vi "Main.vi"() -> ()   [LabVIEW 2020]
doc: "This Continuous Measurement sample project is based on the Queued Message Handler template.\n\nThe Event Handling Loop generates messages based on user interface actions.\n\nThe Message Handling Loop processes messages generated by the Event Handling Loop, or by other messages. There are also Acquisition and Logging message handling loop subVIs, and a chart updating loop."
uses:
  controls/UI Data.ctl
  Modbus/Modbus All Data.ctl
  Modbus/Modbus PLC Data All.ctl
  Modbus/Modbus FVIR Control.ctl
  Modbus/Modbus LDO Control.ctl
  WritingDataFile/Data to Save.ctl
  Modbus/Modbus Gas Meter Data.ctl
  Drivers/Alicat LabVIEW Drivers 2v1/Sub-VIs/Data Cluster.ctl
  Drivers/Alicat LabVIEW Drivers 2v1/Sub-VIs/Units of Measure.ctl
  Drivers/Inficon Transmitter/Type Definitions/Inficon Data.ctl
  support/Event Booleans.ctl
  support/Message Queue/Enqueue Message (Single).vi
  <vilib>/Utility/error.llb/Error Cluster From Error Code.vi
  <vilib>/ErrorRing/Error Ring.xnode
  support/User Event - Stop/User Event - Stop.lvlib
  support/Message Queue/Message Queue.lvlib
  Modbus/Modbus.lvlib
  ReadingDataFile/ReadingDataFile.lvlib
  WritingDataFile/WritingDataFile.lvlib
panel:
  out "Message Loop":string[](array[string])
  out "Numeric 2":i32
  out "Numeric":i32
  in  "Tab Control":enum32{"FVIR", "LDO", "Administrator"}(tab)
  out "Actuator spill can is going to Work Pos - FVIR":bool
  out "Actuator spill can is going to Home Pos - FVIR":bool
  out "Actuator mannequin is going to Work Pos - FVIR":bool
  out "Actuator mannequin is going to Home Pos - FVIR":bool
  out "Error - FVIR":bool caption="Error"
  out "Status for error - FVIR":string caption="Error status for FVIR"
  in  "Move mannequin - Go to Work Pos":bool
  in  "Move mannequin - Go to Home Pos":bool
  in  "Spill can - Go to Work Pos":bool
  in  "Spill can - Go to Home Pos":bool
  out "Start recording data - FVIR":bool
  out "Test chamber is in sequence - FVIR":bool
  out "Can is spilling - FVIR":bool
  out "Mannequin is moving - FVIR":bool
  in  "Select test case":i32(listbox)
  in  "Stop Test Case FVIR":bool
  in  "Start Test Case FVIR":bool
  in  "Time Delay of Change direction of Mannequin Actuators":u16=1000
  in  "Number of Mannequin Movement":u16=3
  in  "Water Outlet Proportional Valve EPV-312B":u16=3
  in  "Water Temperature Intellifaucet DRK375":u16=70
  in  "Water Flow Intellifaucet DRK375":u16=15
  in  "Time Pause Between Next Mannequin Sequence":u16=60
  in  "Send parameters to PLC FVIR":bool
  in  "Water Outlet Valve Close FVIR":bool
  in  "Water Outlet Valve Open FVIR":bool
  in  "Gas Solenoid Valve Close FVIR":bool
  in  "Gas Solenoid Valve Open FVIR":bool
  in  "Water Inlet Valve Close FVIR":bool
  in  "Water Inlet Valve Open FVIR":bool
  in  "Water Flow Intellifaucet DRK375 Close FVIR":bool
  in  "Water Flow Intellifaucet DRK375 Open FVIR":bool
  out "Temperatures - FVIR":string[][](array[string])
  out "Sensors - FVIR":string[][](array[string])
  in  "Water Outlet Flow Proportional Valve EPV-312B Close FVIR":bool
  in  "Water Outlet Flow Proportional Valve EPV-312B Open FVIR":bool
  out "Water Outlet Flow Proportional - FVIR":bool
  out "Water flow DRK375 is open - FVIR":bool
  out "Gas Solenoid Valuce - FVIR":bool
  out "Water Inlet Valve - FVIR":bool
  out "Water Outlet Valve - FVIR":bool
  out "General status for FVIR":string
  out "Higher than 1.8% butane":bool
  in  "Start":bool
  in  "Stop":bool
  in  "Path to local logfile":path=path "C:/Users/christian.hansen/Desktop/GE Appliance - FVIR/GEA_Labview_FVIR/CH1234dummy.LOG"
  in  "Reset Flow Meter":bool
  in  "Gas Meter Tare Total":bool
  in  "Gas Meter Tare Rate":bool
  out "Data":string[][](array[string])
  in  "Proportioning Valve":dbl(slide) max=100.0 scale=0.0..100.0
  in  "Valve % Open":dbl(slide)=15.0 min=15.0 max=100.0 scale=15.0..100.0
  in  "Temp (°F)":dbl(slide)=32.0 min=32.0 max=203.0 scale=32.0..200.0
  in  "Water Flow Intellifaucet DRK375 Open LDO":bool
  in  "Water Flow Intellifaucet DRK375 Close LDO":bool
  out "Heater ON/OFF - LDO":bool
  out "Oil spray 1.33cc/min - LDO":bool
  out "Oil spray 1.1cc/min - LDO":bool
  out "Oil spray 0.8cc/min - LDO":bool
  out "Burner ON":bool
  out "Start recording data - LDO":bool
  out "Test chamber is in sequence - LDO":bool
  in  "Stop Test Case LDO":bool
  in  "Start Test Case LDO":bool
  in  "Water Outlet Valve Close LDO":bool
  in  "Water Outlet Valve Open LDO":bool
  in  "Water Inlet Valve Close LDO":bool
  in  "Water Inlet Valve Open LDO":bool
  in  "Gas Solenoid Valve Close LDO":bool
  in  "Gas Solenoid Valve Open LDO":bool
  in  "Oil Spray 0.8 cc/min Close":bool
  in  "Oil Spray 0.8 cc/min Open":bool
  in  "Oil Spray 1.1 cc/min Close":bool
  in  "Oil Spray 1.1 cc/min Open":bool
  in  "Oil Spray 1.33 cc/min Close":bool
  in  "Oil Spray 1.33 cc/min Open":bool
  in  "Heater OFF":bool
  in  "Heater ON":bool
  out "Water Outlet Flow Proportional - LDO":bool
  out "Water flow DRK375 is open - LDO":bool
  out "Gas Solenoid Valuce - LDO":bool
  out "Water Inlet Valve - LDO":bool
  out "Water Outlet Valve - LDO":bool
  in  "Temp/Flow PID Selector":bool=TRUE
  in  "Precondition Purge Gallons":u16=200 caption="Precondition Purge Time (Sec)"
  in  "Output Flow Rate Target (Automated Test)":dbl=0.75 caption="Output Flow Target (Automated Test)"
  in  "Pilot Rate (BTU/hr)":dbl=600.0
  in  "Output Temperature Target (Automated Test)":dbl=135.0
  out "FVIR PLC lifebit":bool
  out "Labview lifebit":bool
  in  "Send parameters to PLC LDO":bool
  in  "Burner cycle 1 to 10 - Duty cycle ON (default 55 min.)":u16=55 caption="Burner cycle 1 to 10 - Duty cycle ON"
  in  "Burner cycle 1 to 10 - Duty cycle OFF (default 5 min.)":u16=5 caption="Burner cycle 1 to 10 - Duty cycle OFF"
  in  "Burner cycle 11 to 12 - Duty cycle ON (default 235 min.)":u16=235 caption="Burner cycle 11 to 12 - Duty cycle ON"
  in  "Burner cycle 11 to 12 - Duty cycle OFF (default 5 min.)":u16=5 caption="Burner cycle 11 to 12 - Duty cycle OFF"
  in  "Burner cycle 13 to end - Duty cycle ON (default 55 min.)":u16=55 caption="Burner cycle 13 to end - Duty cycle ON"
  in  "Burner cycle 13 to end - Duty cycle OFF (default 5 min.)":u16=5 caption="Burner cycle 13 to end - Duty cycle OFF"
  in  "Oil 1st sequence ON (default 5 min.)":u16=5 caption="Oil 1st sequence ON"
  in  "Oil 1st sequence OFF (default 5 min.)":u16=25 caption="Oil 1st sequence OFF"
  in  "All subsequent sequence ON (default 3 min.)":u16=3 caption="All subsequent sequence ON"
  in  "All subsequent sequence OFF (default 27 min.)":u16=27 caption="All subsequent sequence OFF"
  in  "Oil spray preconditioning period ON (default 10 min.)":u16=10 caption="Oil spray preconditioning period ON"
  in  "Oil spray preconditioning period OFF  (default 20 min.)":u16=20 caption="Oil spray preconditioning period OFF"
  out "General status for LDO":string
  out "Status for error - LDO":string caption="Error status for LDO"
  out "Error - LDO":bool caption="Error"
  in  "PLC IP address":string="10.2.0.11"
  in  "Inficon IP Address":string="192.168.1.32"
  in  "Ultramat 23":refnum<visa-resource-name>="COM13"
  # "FVIR and LDO:Swap the data, i.e. 28-10-2021 --> 2021-10-28. --> Lets test this first to see the currents PC timeformat. \nAll data is in the file now. Also the status of LEDs and what Labview is sending --> A lot of redundant info here. What from \nLabview --> PLC should be recorded?"
  # "FVIR: Missing implementation: Getting the glas flow rate, SQRH. CO, CO2 and O2 from the VI's from GEA"
  # "FVIR"
  # "Main control"
  # "Actuator spill can is going to Work Pos"
  # "Actuator spill can is going to Home Pos"
  # "Actuator mannequin is going to Work Pos"
  # "Actuator mannequin is going to Home Pos"
  # "Automatic mode"
  # "Start recording FVIR data"
  # "Test chamber is in sequence"
  # "Can is spilling"
  # "Mannequin is moving"
  # "Water Outlet Valve"
  # "Gas Solenoid Valve"
  # "Water Inlet Valve"
  # "Water Flow Intellifaucet DRK375"
  # "Water Outlet Flow Proportional EPV-312B"
  # "Water Outlet Flow Proportional is open"
  # "Water flow DRK375 is open"
  # "Gas Solenoid is open"
  # "Water Inlet is open"
  # "Water Outlet is open"
  # "Status of valves"
  # "Manual mode"
  # "Temperature from textfile - 4 channels"
  # "Status of actuators"
  # "Values from FVIR sensors"
  # "Status of chamber"
  # "Changing parameters to PLC"
  # "Main control"
  # "Manual mode"
  # "Status of devices"
  # "Status of chamber"
  # "Status of valves"
  # "Water Flow Intellifaucet DRK375"
  # "Gas Meter"
  # "Rotary Actuator"
  # "Oil spray 1.33cc/min"
  # "Oil spray 1.1cc/min"
  # "Oil spray 0.8cc/min"
  # "Start recording LDO data"
  # "Test chamber is in sequence"
  # "Automatic mode"
  # "Start and stop LDO test"
  # "Water Outlet Valve"
  # "Water Inlet Valve"
  # "Gas Solenoid Valve"
  # "Oil spray at 0.8 cc/min"
  # "Oil spray at 1.1 cc/min"
  # "Oil spray at 1.33 cc/min"
  # "Heater"
  # "Water Outlet Flow Proportional is open"
  # "Water flow DRK375 is open"
  # "Gas Solenoid is open"
  # "Water Inlet is open"
  # "Water Outlet is open"
  # "LDO Parameters -"
  # "Changing parameters to PLC"
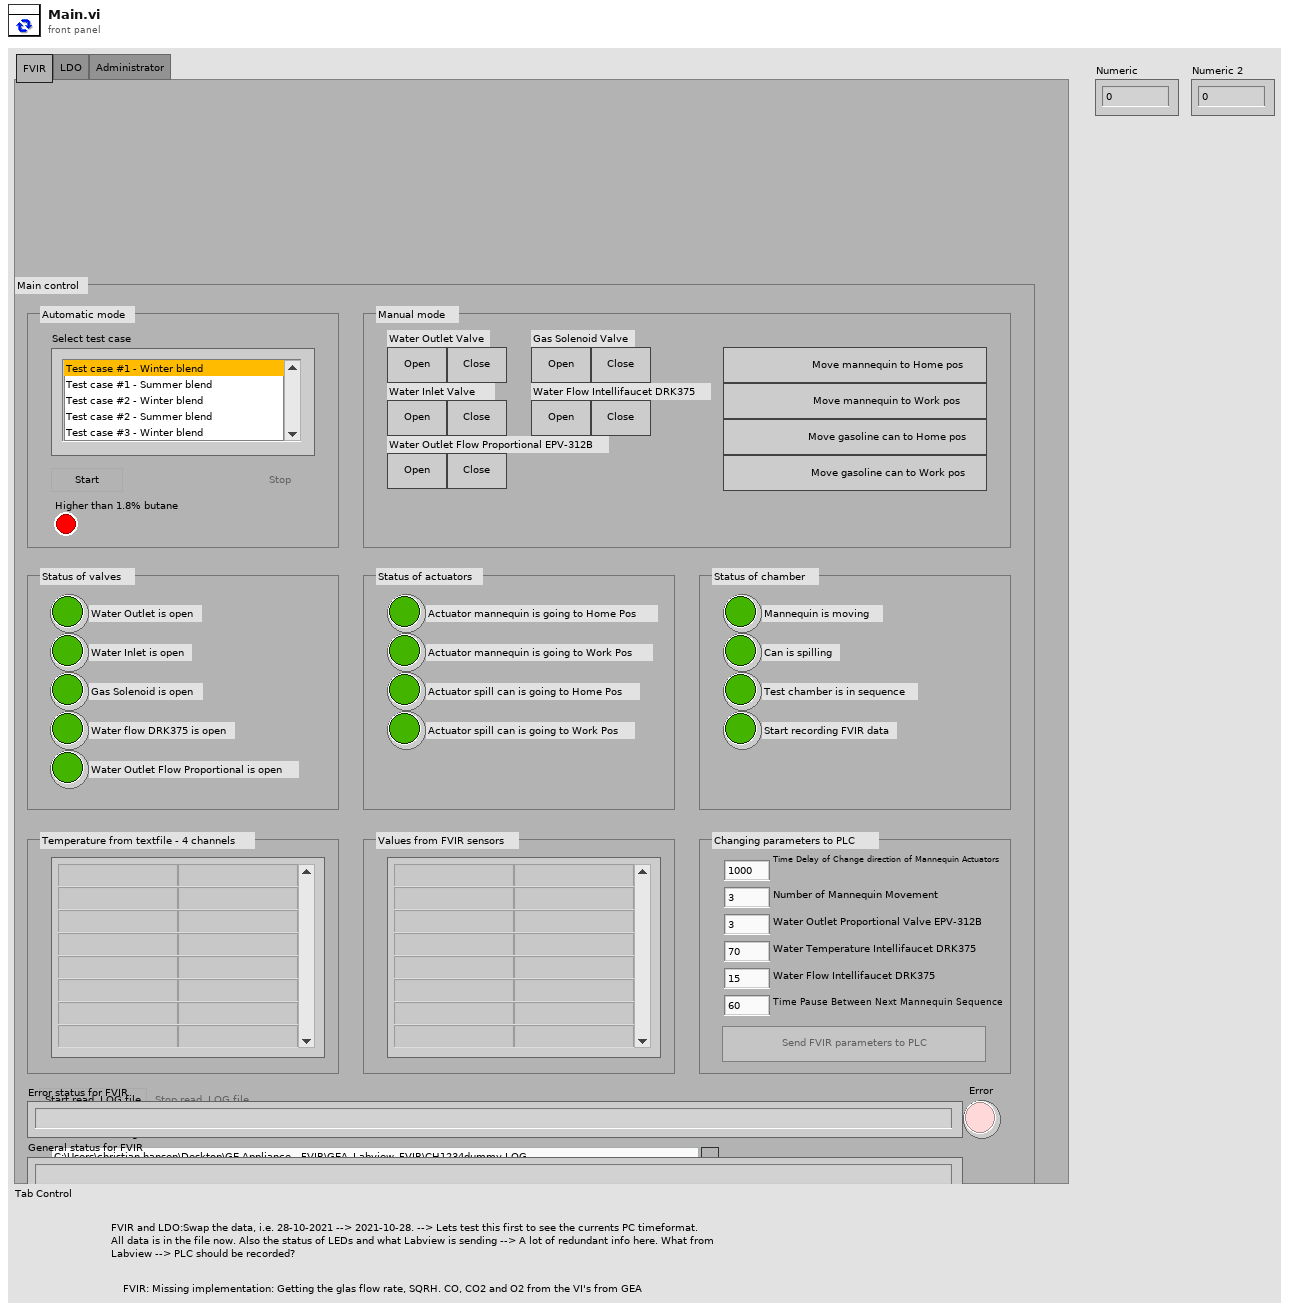
[diagram p1: front panel]
types:
  T1 = typedef "Event Booleans.ctl" = cluster{"Burner ON":bool, "0.8 ml Bool":bool, "1.1 Bool":bool, "1.33 Bool":bool}
  T2 = typedef "Modbus All Data.ctl" = cluster{"PLC Data Out":T3, "Gas Data":T7, "Inficon Data Input":T10, "Ultramat 23":string[][]}
  T3 = typedef "Modbus PLC Data All.ctl" = cluster{"FVIR Data Input":T4, "LDO Control Input":T5, "PLC Input Registers":u16[], "Data to Save":T6}
  T4 = typedef "Modbus FVIR Control.ctl" = cluster{"Spare 15":bool, "Spare 14":bool, "Actuator mannequin is going to Work Pos - FVIR":bool, "Actuator mannequin is going to Home Pos - FVIR":bool, "Test chamber is in sequence - FVIR ":bool, "Water flow DRK375 is open - FVIR":bool, "Gas Solenoid Valve - FVIR":bool, "Water Inlet Valve - FVIR":bool, "Water Outlet Flow Proportional - FVIR":bool, "Start recording data - FVIR":bool, "Actuator spill can is going to Work Pos - FVIR":bool, "Actuator spill can is going to Home Pos - FVIR":bool, "Water Outlet Valve - FVIR":bool, "Can is spilling - FVIR":bool, "Mannequin is moving - FVIR":bool, "FVIR PLC lifebit":bool, "Status for Error - FVIR":string, "Error-FVIR":bool, "Sensors -FVIR":string[][]}
  T5 = typedef "Modbus LDO Control.ctl" = cluster{"LDO PLC Life Bit":bool, "Start recording data - LDO":bool, "Spare 1":bool, "Water Outlet Valve - LDO":bool, "Water Inlet Valve - LDO":bool, "Gas Solenoid Valve - LDO":bool, "Water flow DRK375 is open - LDO":bool, "Test chamber is in sequence - LDO":bool, "Oil spray 0.8cc/min - LDO":bool, "Oil spray 1.1cc/min - LDO":bool, "Oil spray 1.33cc/min - LDO":bool, "Heater ON/OFF - LDO":bool, "Water Outlet Flow Proportional - LDO":bool, "Spare 2":bool, "Spare 3":bool, "Spare 4":bool, "Status for error - LDO":string, "Error - LDO":bool, "Sensor Data":string[][]}
  T6 = typedef "Data to Save.ctl" = cluster{"LDO Full Data":string[][], "FVIR Full Data":string[][], "Test Case - FVIR":string, "Test Case - LDO":string}
  T7 = typedef "Modbus Gas Meter Data.ctl" = cluster{"Data Cluster":T8, "Units of Measure Input":T9, "Header Array":string[]}
  T8 = typedef "Data Cluster.ctl" = cluster{"Absolute Pressure":dbl, "Gauge/Diff. Pressure":dbl, "Barometric Pressure":dbl, "Temperature":dbl, "Volumetric Flow":dbl, "Mass Flow":dbl, "Setpoint":dbl, "Valve Drive":dbl, "Totalizer":dbl, "[hr]":dbl, "[min]":dbl, "[sec]":dbl, "Totalizer Average Flow":dbl, "Totalizer Peak Flow":dbl, "Gas selected":string}
  T9 = typedef "Units of Measure.ctl" = cluster{"Abs. Pressure":string, "Gauge/Diff. Press.":string, "Barometric Press.":string, "Temperature":string, "Volume":string, "Mass":string, "Setpoint":string, "Valve Drive":string, "Totalizer":string, "Tot. Timer":string, "Tot. Avg. Flow":string, "Tot. Peak Flow":string}
  T10 = typedef "Inficon Data.ctl" = cluster{"Gross Heating Value, Vol (Real, Dry)":dbl, "Nitrogen Component Normalized Mole % (Dry)":dbl, "Methane Component Normalized Mole % (Dry)":dbl, "Carbon Dioxide Component Normalized Mole % (Dry)":dbl, "Ethane Component Normalized Mole % (Dry)":dbl, "Propane Component Normalized Mole % (Dry)":dbl, "i-Pentane Component Normalized Mole % (Dry)":dbl, "i-Butane Component Normalized Mole % (Dry)":dbl, "n-Butane Component Normalized Mole % (Dry)":dbl, "n-Pentane Component Normalized Mole % (Dry)":dbl, "Hexane Component Normalized Mole % (Dry)":dbl, "Heptane Component Normalized Mole % (Dry)":dbl, "Gross Wobbe Index, Real(Dry)":dbl, "Relative Density, Real(Dry)":dbl, "Propylene Component Normalized Mole % (Dry)":dbl, "C4 Olefins Component Normalized Mole % (Dry)":dbl, "Water Component Normalized Mole % (Dry)":dbl}
  T11 = typedef "UI Data.ctl" = cluster{"Start Ref":refnum<vi>, "Stop Ref":refnum<vi>, "Exit Ref":refnum<vi>, "Status Ref":refnum<vi>, "Connect Ref":refnum<vi>, "Disconnect Ref":refnum<vi>, "Spill can Home pos Ref":refnum<vi>, "Spill can Work pos Ref":refnum<vi>, "Move Mannequin Home pos Ref":refnum<vi>, "Move Mannequin Work pos Ref":refnum<vi>, "Start test case FVIR Ref":refnum<vi>, "Water Outlet Valve Open FVIR Ref":refnum<vi>, "Water Inlet Valve Open FVIR Ref":refnum<vi>, "Gas Solenoid Valve Open FVIR Ref":refnum<vi>, "Water Flow Open FVIR Ref":refnum<vi>, "Listbox Ref":refnum<vi>, "Stop test case FVIR Ref":refnum<vi>, "Water Outlet Valve Close FVIR Ref":refnum<vi>, "Water Inlet Valve Close FVIR Ref":refnum<vi>, "Gas Solenoid Valve Close FVIR Ref":refnum<vi>, "Water Flow Close FVIR Ref":refnum<vi>, "Send Param to PLC FVIR Ref":refnum<vi>, "Water Flow Prop Open FVIR Ref":refnum<vi>, "Water Flow Prop Close FVIR Ref":refnum<vi>, "Start test case LDO Ref":refnum<vi>, "Stop test case LDO Ref":refnum<vi>, "Water Outlet Valve Open LDO Ref":refnum<vi>, "Water Outlet Valve Close LDO Ref":refnum<vi>, "Water Inlet Valve Open LDO Ref":refnum<vi>, "Water Inlet Valve Close LDO Ref":refnum<vi>, "Gas Solenoid Valve Open LDO Ref":refnum<vi>, "Gas Solenoid Valve Close LDO Ref":refnum<vi>, "Water Flow Open LDO Ref":refnum<vi>, "Water Flow Close LDO Ref":refnum<vi>, "Water Flow Prop Open LDO Ref":refnum<vi>, "Water Flow Prop Close LDO Ref":refnum<vi>, "Oil spray 0.8cc/min Open Ref":refnum<vi>, "Oil spray 0.8cc/min Close Ref":refnum<vi>, "Oil spray 1.1cc/min Open Ref":refnum<vi>, "Oil spray 1.1cc/min Close Ref":refnum<vi>, "Oil spray 1.33cc/min Open Ref":refnum<vi>, "Oil spray 1.33cc/min Close Ref":refnum<vi>, "Heater ON Ref":refnum<vi>, "Heater OFF Ref":refnum<vi>, "Send Param to PLC LDO Ref":refnum<vi>}
  T12 = typedef "Message Queue.lvlib/All Message Queues.ctl" = cluster{"UI":refnum<queue>, "Modbus":refnum<queue>, "Watchdog":refnum<queue>, "ReadDataFile":refnum<queue>, "DataScanning":refnum<queue>, "WriteDataFile":refnum<queue>, "WatchdogWriteFile":refnum<queue>, "OilMachine":refnum<queue>, "Alicat_GasMeter":refnum<queue>, "Inficon":refnum<queue>, "Ultramat 23":refnum<queue>}
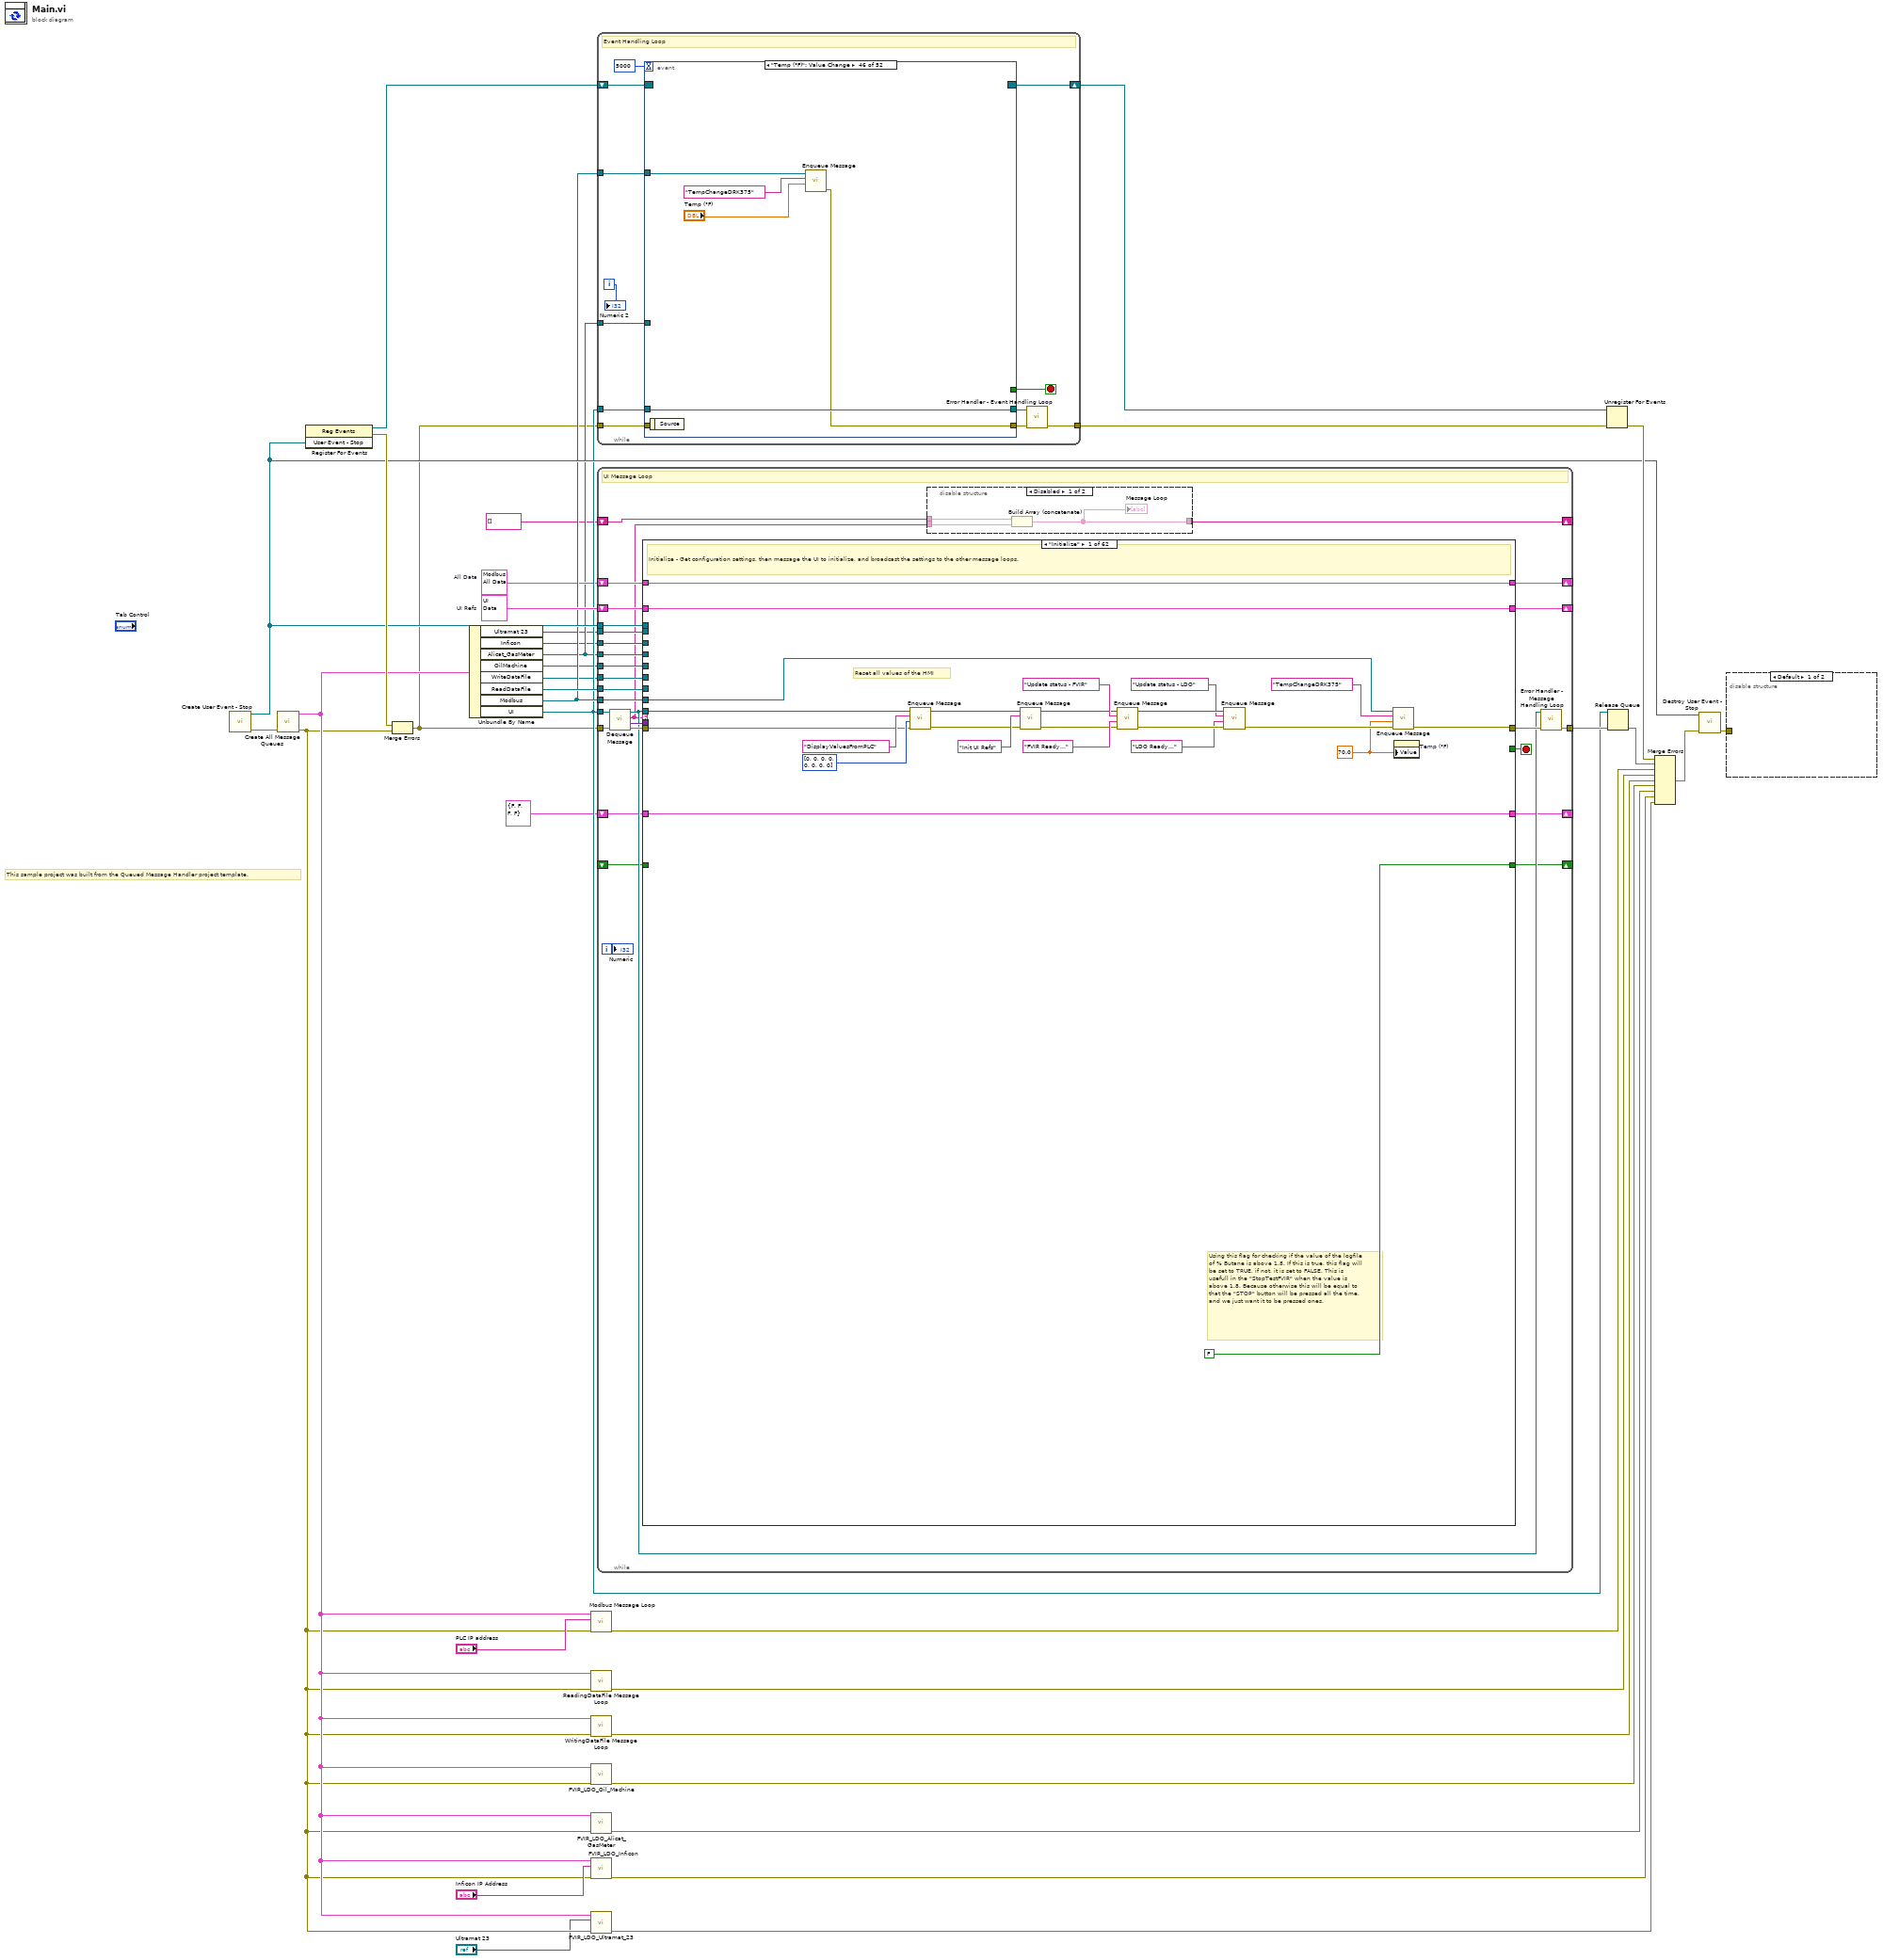
[diagram p0: block diagram]
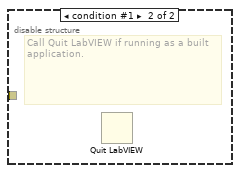
[diagram p2: hidden frame]
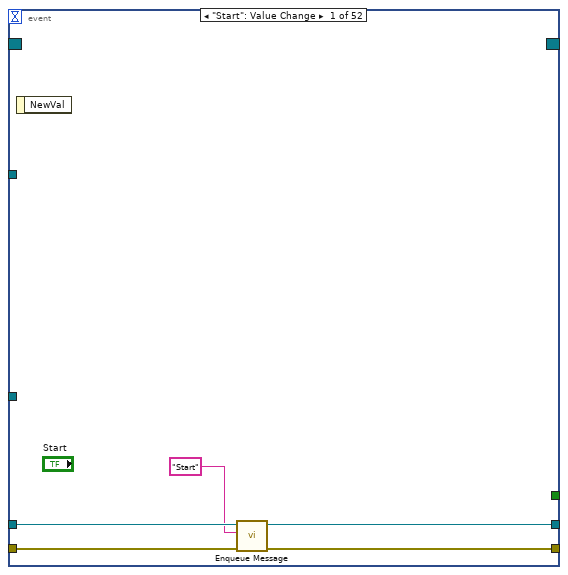
[diagram p3: hidden frame]
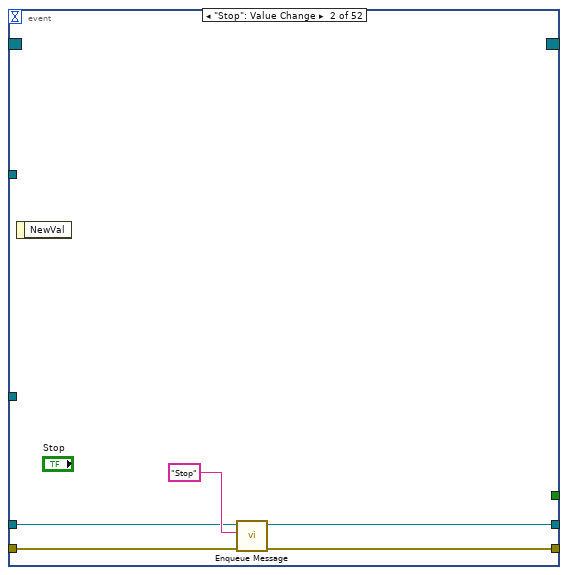
[diagram p4: hidden frame]
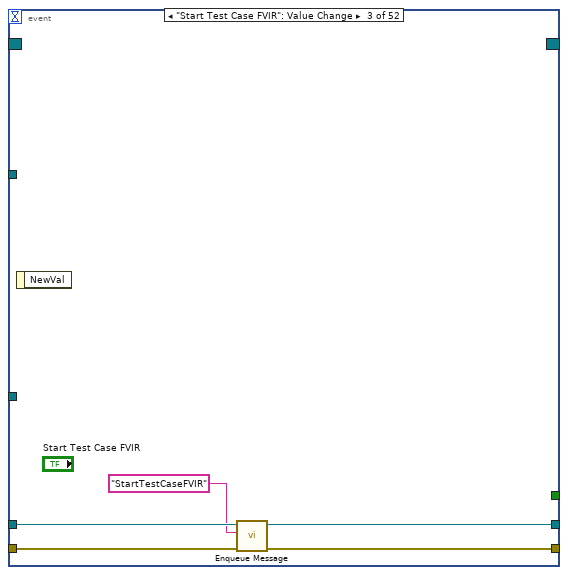
[diagram p5: hidden frame]
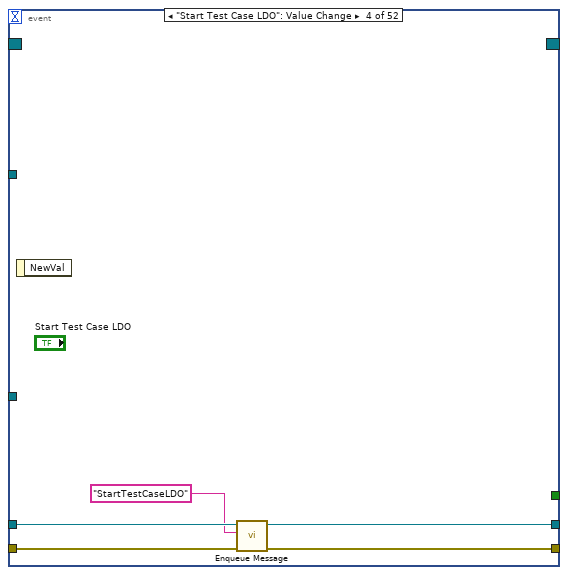
[diagram p6: hidden frame]
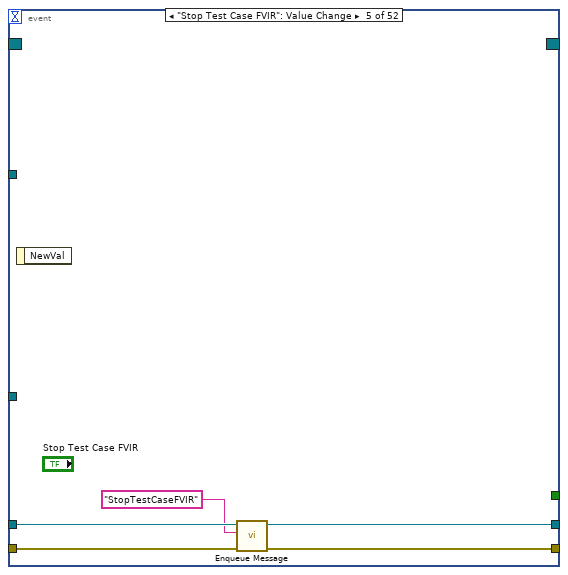
[diagram p7: hidden frame]
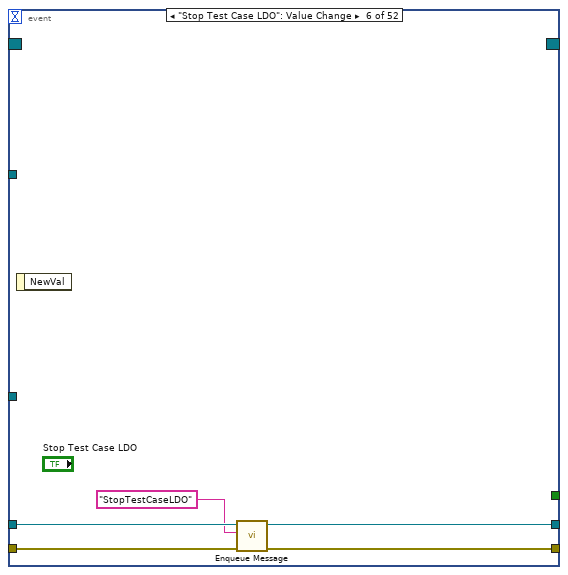
[diagram p8: hidden frame]
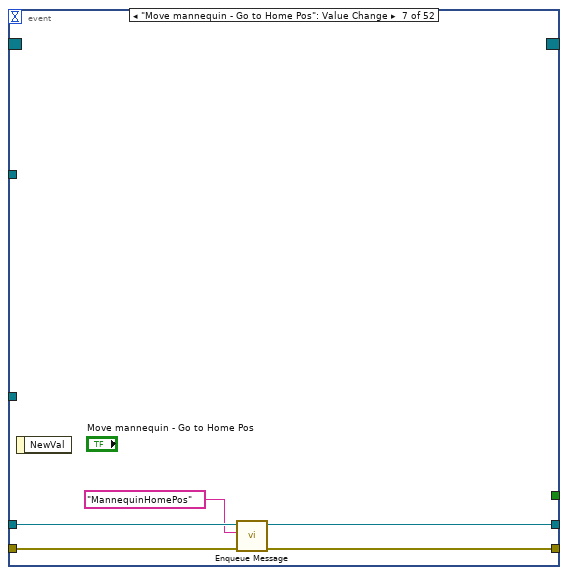
[diagram p9: hidden frame]
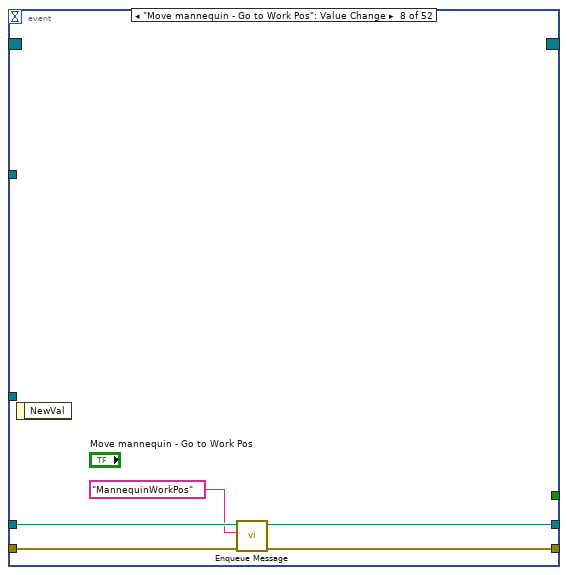
[diagram p10: hidden frame]
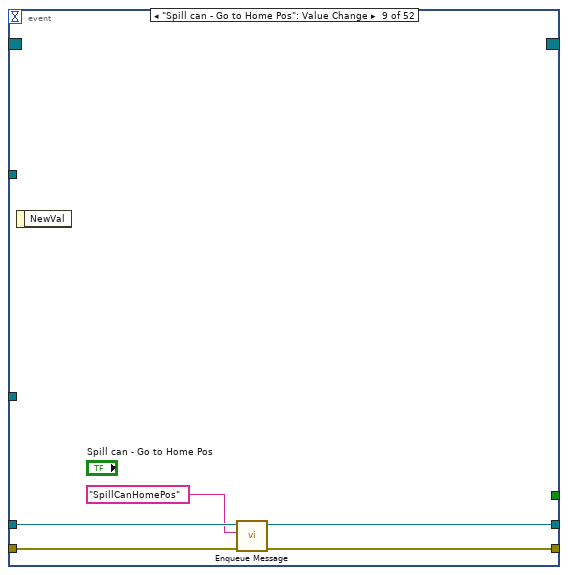
[diagram p11: hidden frame]
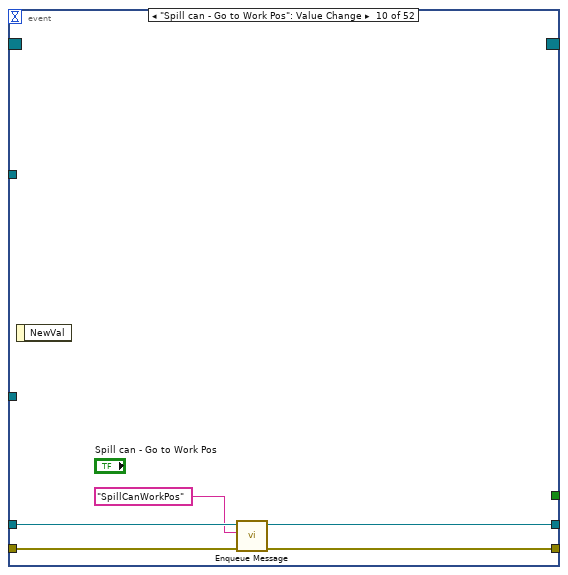
[diagram p12: hidden frame]
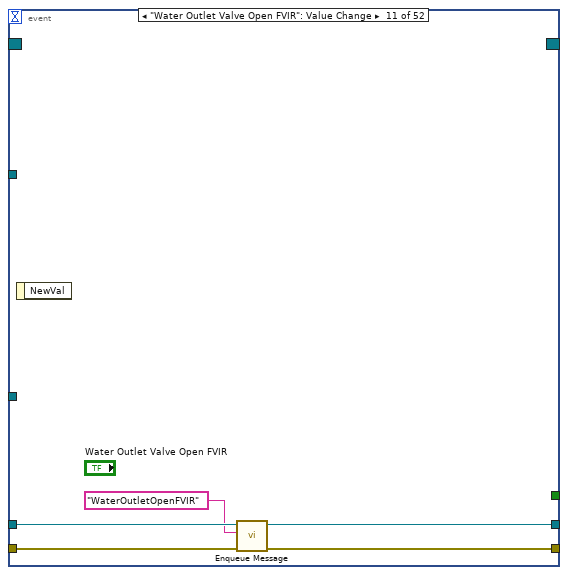
[diagram p13: hidden frame]
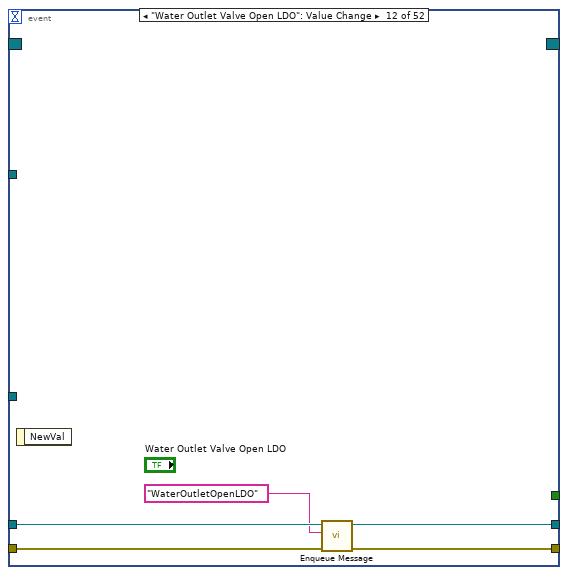
[diagram p14: hidden frame]
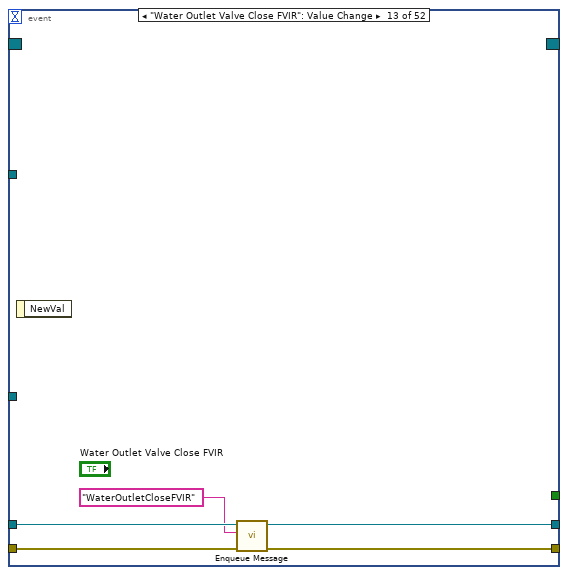
[diagram p15: hidden frame]
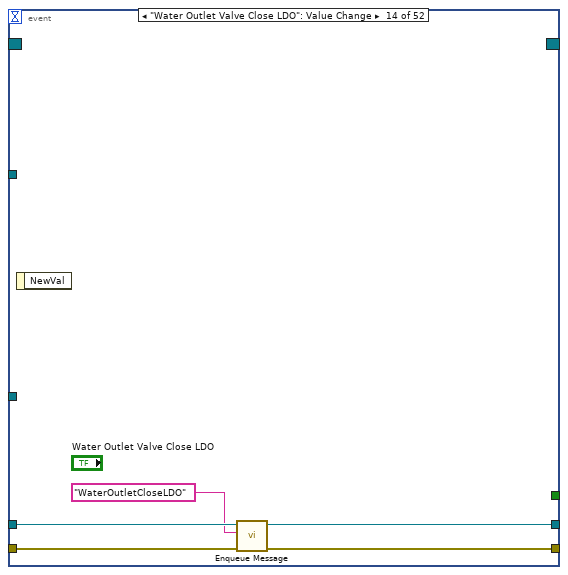
[diagram p16: hidden frame]
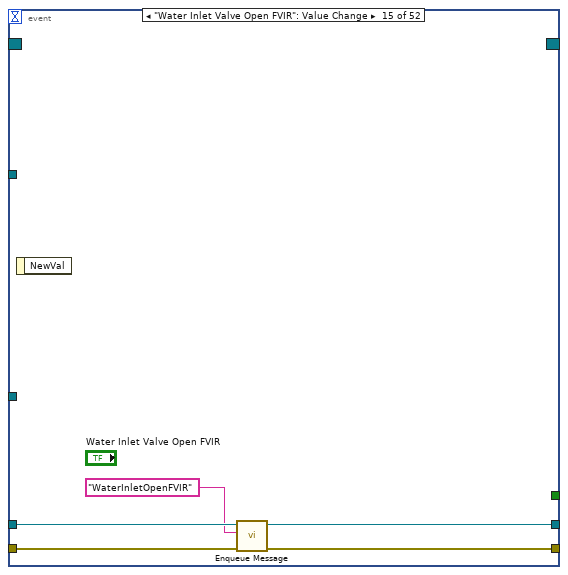
[diagram p17: hidden frame]
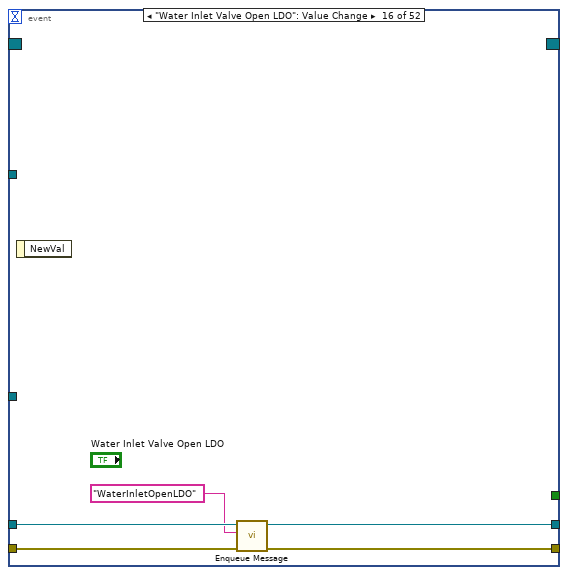
[diagram p18: hidden frame]
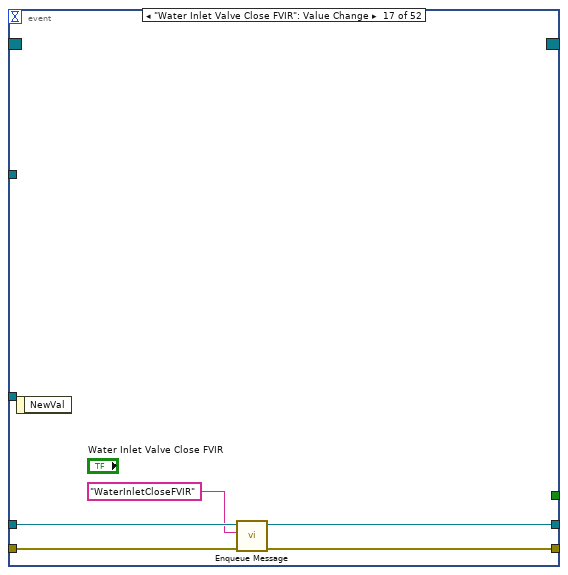
[diagram p19: hidden frame]
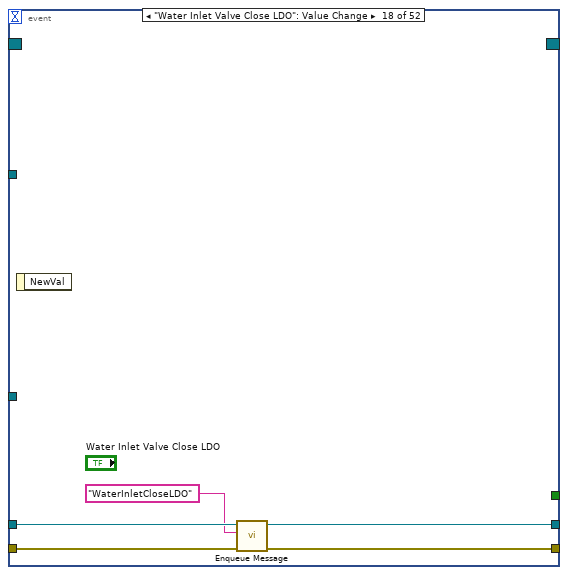
[diagram p20: hidden frame]
diagram:
  w15 = T2 {"PLC Data Out"={"FVIR Data Input"={"Spare 15"=FALSE, "Spare 14"=FALSE, "Actuator mannequin is going to Work Pos - FVIR"=FALSE, "Actuator mannequin is going to Home Pos - FVIR"=FALSE, "Test chamber is in sequence - FVIR "=FALSE, "Water flow DRK375 is open - FVIR"=FALSE, "Gas Solenoid Valve - FVIR"=FALSE, "Water Inlet Valve - FVIR"=FALSE, "Water Outlet Flow Proportional - FVIR"=FALSE, "Start recording data - FVIR"=FALSE, "Actuator spill can is going to Work Pos - FVIR"=FALSE, "Actuator spill can is going to Home Pos - FVIR"=FALSE, "Water Outlet Valve - FVIR"=FALSE, "Can is spilling - FVIR"=FALSE, "Mannequin is moving - FVIR"=FALSE, "FVIR PLC lifebit"=FALSE, "Status for Error - FVIR"="", "Error-FVIR"=FALSE, "Sensors -FVIR"=[]}, "LDO Control Input"={"LDO PLC Life Bit"=FALSE, "Start recording data - LDO"=FALSE, "Spare 1"=FALSE, "Water Outlet Valve - LDO"=FALSE, "Water Inlet Valve - LDO"=FALSE, "Gas Solenoid Valve - LDO"=FALSE, "Water flow DRK375 is open - LDO"=FALSE, "Test chamber is in sequence - LDO"=FALSE, "Oil spray 0.8cc/min - LDO"=FALSE, "Oil spray 1.1cc/min - LDO"=FALSE, "Oil spray 1.33cc/min - LDO"=FALSE, "Heater ON/OFF - LDO"=FALSE, "Water Outlet Flow Proportional - LDO"=FALSE, "Spare 2"=FALSE, "Spare 3"=FALSE, "Spare 4"=FALSE, "Status for error - LDO"="", "Error - LDO"=FALSE, "Sensor Data"=[]}, "PLC Input Registers"=[], "Data to Save"={"LDO Full Data"=[], "FVIR Full Data"=[], "Test Case - FVIR"="", "Test Case - LDO"=""}}, "Gas Data"={"Data Cluster"={"Absolute Pressure"=0.0, "Gauge/Diff. Pressure"=0.0, "Barometric Pressure"=0.0, "Temperature"=0.0, "Volumetric Flow"=0.0, "Mass Flow"=0.0, "Setpoint"=0.0, "Valve Drive"=0.0, "Totalizer"=0.0, "[hr]"=0.0, "[min]"=0.0, "[sec]"=0.0, "Totalizer Average Flow"=0.0, "Totalizer Peak Flow"=0.0, "Gas selected"=""}, "Units of Measure Input"={"Abs. Pressure"="", "Gauge/Diff. Press."="", "Barometric Press."="", "Temperature"="", "Volume"="", "Mass"="", "Setpoint"="", "Valve Drive"="", "Totalizer"="", "Tot. Timer"="", "Tot. Avg. Flow"="", "Tot. Peak Flow"=""}, "Header Array"=[]}, "Inficon Data Input"={"Gross Heating Value, Vol (Real, Dry)"=0.0, "Nitrogen Component Normalized Mole % (Dry)"=0.0, "Methane Component Normalized Mole % (Dry)"=0.0, "Carbon Dioxide Component Normalized Mole % (Dry)"=0.0, "Ethane Component Normalized Mole % (Dry)"=0.0, "Propane Component Normalized Mole % (Dry)"=0.0, "i-Pentane Component Normalized Mole % (Dry)"=0.0, "i-Butane Component Normalized Mole % (Dry)"=0.0, "n-Butane Component Normalized Mole % (Dry)"=0.0, "n-Pentane Component Normalized Mole % (Dry)"=0.0, "Hexane Component Normalized Mole % (Dry)"=0.0, "Heptane Component Normalized Mole % (Dry)"=0.0, "Gross Wobbe Index, Real(Dry)"=0.0, "Relative Density, Real(Dry)"=0.0, "Propylene Component Normalized Mole % (Dry)"=0.0, "C4 Olefins Component Normalized Mole % (Dry)"=0.0, "Water Component Normalized Mole % (Dry)"=0.0}, "Ultramat 23"=[]}  # All Data
  w31 = T11 {"Start Ref"=refnum, "Stop Ref"=refnum, "Exit Ref"=refnum, "Status Ref"=refnum, "Connect Ref"=refnum, "Disconnect Ref"=refnum, "Spill can Home pos Ref"=refnum, "Spill can Work pos Ref"=refnum, "Move Mannequin Home pos Ref"=refnum, "Move Mannequin Work pos Ref"=refnum, "Start test case FVIR Ref"=refnum, "Water Outlet Valve Open FVIR Ref"=refnum, "Water Inlet Valve Open FVIR Ref"=refnum, "Gas Solenoid Valve Open FVIR Ref"=refnum, "Water Flow Open FVIR Ref"=refnum, "Listbox Ref"=refnum, "Stop test case FVIR Ref"=refnum, "Water Outlet Valve Close FVIR Ref"=refnum, "Water Inlet Valve Close FVIR Ref"=refnum, "Gas Solenoid Valve Close FVIR Ref"=refnum, "Water Flow Close FVIR Ref"=refnum, "Send Param to PLC FVIR Ref"=refnum, "Water Flow Prop Open FVIR Ref"=refnum, "Water Flow Prop Close FVIR Ref"=refnum, "Start test case LDO Ref"=refnum, "Stop test case LDO Ref"=refnum, "Water Outlet Valve Open LDO Ref"=refnum, "Water Outlet Valve Close LDO Ref"=refnum, "Water Inlet Valve Open LDO Ref"=refnum, "Water Inlet Valve Close LDO Ref"=refnum, "Gas Solenoid Valve Open LDO Ref"=refnum, "Gas Solenoid Valve Close LDO Ref"=refnum, "Water Flow Open LDO Ref"=refnum, "Water Flow Close LDO Ref"=refnum, "Water Flow Prop Open LDO Ref"=refnum, "Water Flow Prop Close LDO Ref"=refnum, "Oil spray 0.8cc/min Open Ref"=refnum, "Oil spray 0.8cc/min Close Ref"=refnum, "Oil spray 1.1cc/min Open Ref"=refnum, "Oil spray 1.1cc/min Close Ref"=refnum, "Oil spray 1.33cc/min Open Ref"=refnum, "Oil spray 1.33cc/min Close Ref"=refnum, "Heater ON Ref"=refnum, "Heater OFF Ref"=refnum, "Send Param to PLC LDO Ref"=refnum}  # UI Refs
  # "This sample project was built from the Queued Message Handler project template."
  n1 = call "Create User Event - Stop.vi"() -> ("error out"=w34:errorcluster, "User Event - Stop"=w26:refnum<user-event>)  [unwired: 10 in]
  n2 = call "Create All Message Queues.vi"("error in (no error)"=w34) -> ("error out"=w10:errorcluster, "Message Queues out"=w11:T12)  [unwired: 9 in]
  n3 = register-events(w26) -> (reference out=w28:refnum<event-registration>, error out=w27:errorcluster)  [unwired: 2 in]
  n4 = Merge Errors(w27, w10) -> (w2:errorcluster)
  n5 = Unbundle By Name(w11) -> ("Ultramat 23"=w5:refnum<queue>, "Inficon"=w13:refnum<queue>, "Alicat_GasMeter"=w14:refnum<queue>, "OilMachine"=w17:refnum<queue>, "WriteDataFile"=w1:refnum<queue>, "ReadDataFile"=w25:refnum<queue>, "Modbus"=w24:refnum<queue>, "UI"=w19:refnum<queue>)
  n6 = call "Modbus Message Loop.vi"("Message Queues in"=w11, "PLC IP address"="PLC IP address", "error in (no error)"=w10) -> ("error out"=w23:errorcluster)  [unwired: 7 in]
  n7 = call "ReadingDataFile Message Loop.vi"("error in (no error)"=w10, "Message Queues"=w11) -> ("error out"=w22:errorcluster)  [unwired: 7 in, 1 out]
  n8 = call "WritingDataFile Message Loop.vi"("error in (no error)"=w10, "Message Queues"=w11) -> ("error out"=w21:errorcluster)  [unwired: 9 in]
  n9 = call "FVIR_LDO_Oil_Machine.vi"("error in"=w10, "Message Queues"=w11) -> ("error out"=w18:errorcluster)  [unwired: 9 in]
  n10 = call "FVIR_LDO_Alicat_GasMeter.vi"("error in"=w10, "Message Queues"=w11) -> ("error out"=w9:errorcluster)  [unwired: 9 in]
  n11 = call "FVIR_LDO_Inficon.vi"("error in"=w10, "Remote IP Address"="Inficon IP Address", "Message Queues"=w11) -> ("error out"=w8:errorcluster)  [unwired: 8 in]
  n12 = call "FVIR_LDO_Ultramat_23.vi"("error in"=w10, "VISA resource name"="Ultramat 23", "Message Queues"=w11) -> ("error out"=w7:errorcluster)  [unwired: 8 in]
  n13 = while {
    tunnel: w19 -> [w47]
    tunnel: [w44] -> w35
    shift-right: [w46] -> w32
    shift-left: w28 -> [w48]
    tunnel: w24 -> [w40]
    tunnel: w14 -> [w39]
    tunnel: w2 -> [w37]
    i -> [w38]
    stop <- w45 stop-if-true
    # "Event Handling Loop"
    n14 = event shown="[45] \"Temp (°F)\": Value Change" {
      selector: w48 -> [_ _ _ _ _ _ _ _ _ _ _ _ _ _ _ _ _ _ _ _ _ _ _ _ _ _ _ _ _ _ _ _ _ _ _ _ _ _ _ _ _ _ _ _ _ _ _ _ _ _ _ _]
      dyn-events: [_ _ _ _ _ _ _ _ _ _ _ _ _ _ _ _ _ _ _ _ _ _ _ _ _ _ _ _ _ _ _ _ _ _ _ _ _ _ _ _ _ _ _ _ _ _ _ _ _ _ _ _] -> w46
      timeout: 5000 -> [_ _ _ _ _ _ _ _ _ _ _ _ _ _ _ _ _ _ _ _ _ _ _ _ _ _ _ _ _ _ _ _ _ _ _ _ _ _ _ _ _ _ _ _ _ _ _ _ _ _ _ _]
      tunnel: [_ _ _ _ _ _ _ _ _ _ _ _ _ _ _ _ _ _ _ _ _ _ _ _ _ _ _ _ _ _ _ _ _ _ _ _ _ _ _ _ _ _ _ TRUE ("Discard?") _ _ _ _ _ _ _ _] -> w45
      tunnel: w47 -> [w53 w57 w63 w68 w73 w78 w83 w88 w93 w98 w103 w108 w113 w118 w123 w128 w133 w138 w143 w148 w153 w158 w163 w173 w180 w190 w197 w202 w207 w212 w217 w225 w230 w235 w243 w248 w253 w261 w266 w271 w276 w281 w285 w288 w291 w308 w313 w318 w322 w326 w335 w342]
      tunnel: [w51 w56 w61 w66 w71 w76 w81 w86 w91 w96 w101 w106 w111 w116 w121 w126 w131 w136 w141 w146 w151 w156 w161 w169 w178 w188 w195 w200 w205 w210 w216 w223 w228 w233 w241 w246 w251 w259 w264 w269 w274 w279 w284 w286 w296 w304 w309 w314 w319 w323 w330 w340] -> w43
      tunnel: [w50 w55 w60 w65 w70 w75 w80 w85 w90 w95 w100 w105 w110 w115 w120 w125 w130 w135 w140 w145 w150 w155 w160 w170 w177 w186 w194 w199 w204 w209 w215 w222 w227 w234 w240 w245 w252 w258 w263 w268 w273 w280 w285 w288 w290 w308 w313 w318 w322 w326 w335 w342] -> w42
      tunnel: w40 -> [_ _ _ _ _ _ _ _ _ _ _ _ _ _ _ _ _ _ _ _ _ _ _ _ _ _ _ _ _ _ _ _ _ _ _ _ _ _ _ _ _ _ _ _ _ w306 w311 w316 _ _ w331 w339]
      tunnel: w39 -> [_ _ _ _ _ _ _ _ _ _ _ _ _ _ _ _ _ _ _ _ _ _ _ _ _ _ _ _ _ _ _ _ _ _ _ _ _ _ _ _ _ _ _ _ _ _ _ _ w320 w324 _ _]
      tunnel: w37 -> [w49 w54 w59 w64 w69 w74 w79 w84 w89 w94 w99 w104 w109 w114 w119 w124 w129 w134 w139 w144 w149 w154 w159 w164 w176 w181 w193 w198 w203 w208 w213 w221 w226 w231 w239 w244 w249 w257 w262 w267 w272 w277 w284 w286 w295 _ _ _ _ _ _ _]
      event "Start": Value Change {
        n15 = event-data() -> ()  [unwired: 1 in, 1 out]
        n16 = call-poly "Enqueue Message.vi"("error in (no error)"=w49, "Message"="Start", "Message Queue"=w53) -> ("error out"=w51:errorcluster, "dup Message Queue"=w50:refnum<queue>)  [unwired: 7 in]
      }
      event "Stop": Value Change {
        n17 = event-data() -> ()  [unwired: 1 in, 1 out]
        n18 = call-poly "Enqueue Message.vi"("error in (no error)"=w54, "Message"="Stop", "Message Queue"=w57) -> ("error out"=w56:errorcluster, "dup Message Queue"=w55:refnum<queue>)  [unwired: 7 in]
      }
      event "Start Test Case FVIR": Value Change {
        n19 = event-data() -> ()  [unwired: 1 in, 1 out]
        n20 = call-poly "Enqueue Message.vi"("error in (no error)"=w59, "Message"="StartTestCaseFVIR", "Message Queue"=w63) -> ("error out"=w61:errorcluster, "dup Message Queue"=w60:refnum<queue>)  [unwired: 7 in]
      }
      event "Start Test Case LDO": Value Change {
        n21 = event-data() -> ()  [unwired: 1 in, 1 out]
        n22 = call-poly "Enqueue Message.vi"("error in (no error)"=w64, "Message"="StartTestCaseLDO", "Message Queue"=w68) -> ("error out"=w66:errorcluster, "dup Message Queue"=w65:refnum<queue>)  [unwired: 7 in]
      }
      event "Stop Test Case FVIR": Value Change {
        n23 = event-data() -> ()  [unwired: 1 in, 1 out]
        n24 = call-poly "Enqueue Message.vi"("error in (no error)"=w69, "Message"="StopTestCaseFVIR", "Message Queue"=w73) -> ("error out"=w71:errorcluster, "dup Message Queue"=w70:refnum<queue>)  [unwired: 7 in]
      }
      event "Stop Test Case LDO": Value Change {
        n25 = event-data() -> ()  [unwired: 1 in, 1 out]
        n26 = call-poly "Enqueue Message.vi"("error in (no error)"=w74, "Message"="StopTestCaseLDO", "Message Queue"=w78) -> ("error out"=w76:errorcluster, "dup Message Queue"=w75:refnum<queue>)  [unwired: 7 in]
      }
      event "Move mannequin - Go to Home Pos": Value Change {
        n27 = event-data() -> ()  [unwired: 1 in, 1 out]
        n28 = call-poly "Enqueue Message.vi"("error in (no error)"=w79, "Message"="MannequinHomePos", "Message Queue"=w83) -> ("error out"=w81:errorcluster, "dup Message Queue"=w80:refnum<queue>)  [unwired: 7 in]
      }
      event "Move mannequin - Go to Work Pos": Value Change {
        n29 = event-data() -> ()  [unwired: 1 in, 1 out]
        n30 = call-poly "Enqueue Message.vi"("error in (no error)"=w84, "Message"="MannequinWorkPos", "Message Queue"=w88) -> ("error out"=w86:errorcluster, "dup Message Queue"=w85:refnum<queue>)  [unwired: 7 in]
      }
      event "Spill can - Go to Home Pos": Value Change {
        n31 = event-data() -> ()  [unwired: 1 in, 1 out]
        n32 = call-poly "Enqueue Message.vi"("error in (no error)"=w89, "Message"="SpillCanHomePos", "Message Queue"=w93) -> ("error out"=w91:errorcluster, "dup Message Queue"=w90:refnum<queue>)  [unwired: 7 in]
      }
      event "Spill can - Go to Work Pos": Value Change {
        n33 = event-data() -> ()  [unwired: 1 in, 1 out]
        n34 = call-poly "Enqueue Message.vi"("error in (no error)"=w94, "Message"="SpillCanWorkPos", "Message Queue"=w98) -> ("error out"=w96:errorcluster, "dup Message Queue"=w95:refnum<queue>)  [unwired: 7 in]
      }
      event "Water Outlet Valve Open FVIR": Value Change {
        n35 = event-data() -> ()  [unwired: 1 in, 1 out]
        n36 = call-poly "Enqueue Message.vi"("error in (no error)"=w99, "Message"="WaterOutletOpenFVIR", "Message Queue"=w103) -> ("error out"=w101:errorcluster, "dup Message Queue"=w100:refnum<queue>)  [unwired: 7 in]
      }
      event "Water Outlet Valve Open LDO": Value Change {
        n37 = event-data() -> ()  [unwired: 1 in, 1 out]
        n38 = call-poly "Enqueue Message.vi"("error in (no error)"=w104, "Message"="WaterOutletOpenLDO", "Message Queue"=w108) -> ("error out"=w106:errorcluster, "dup Message Queue"=w105:refnum<queue>)  [unwired: 7 in]
      }
      event "Water Outlet Valve Close FVIR": Value Change {
        n39 = event-data() -> ()  [unwired: 1 in, 1 out]
        n40 = call-poly "Enqueue Message.vi"("error in (no error)"=w109, "Message"="WaterOutletCloseFVIR", "Message Queue"=w113) -> ("error out"=w111:errorcluster, "dup Message Queue"=w110:refnum<queue>)  [unwired: 7 in]
      }
      event "Water Outlet Valve Close LDO": Value Change {
        n41 = event-data() -> ()  [unwired: 1 in, 1 out]
        n42 = call-poly "Enqueue Message.vi"("error in (no error)"=w114, "Message"="WaterOutletCloseLDO", "Message Queue"=w118) -> ("error out"=w116:errorcluster, "dup Message Queue"=w115:refnum<queue>)  [unwired: 7 in]
      }
      event "Water Inlet Valve Open FVIR": Value Change {
        n43 = event-data() -> ()  [unwired: 1 in, 1 out]
        n44 = call-poly "Enqueue Message.vi"("error in (no error)"=w119, "Message"="WaterInletOpenFVIR", "Message Queue"=w123) -> ("error out"=w121:errorcluster, "dup Message Queue"=w120:refnum<queue>)  [unwired: 7 in]
      }
      event "Water Inlet Valve Open LDO": Value Change {
        n45 = event-data() -> ()  [unwired: 1 in, 1 out]
        n46 = call-poly "Enqueue Message.vi"("error in (no error)"=w124, "Message"="WaterInletOpenLDO", "Message Queue"=w128) -> ("error out"=w126:errorcluster, "dup Message Queue"=w125:refnum<queue>)  [unwired: 7 in]
      }
      event "Water Inlet Valve Close FVIR": Value Change {
        n47 = event-data() -> ()  [unwired: 1 in, 1 out]
        n48 = call-poly "Enqueue Message.vi"("error in (no error)"=w129, "Message"="WaterInletCloseFVIR", "Message Queue"=w133) -> ("error out"=w131:errorcluster, "dup Message Queue"=w130:refnum<queue>)  [unwired: 7 in]
      }
      event "Water Inlet Valve Close LDO": Value Change {
        n49 = event-data() -> ()  [unwired: 1 in, 1 out]
        n50 = call-poly "Enqueue Message.vi"("error in (no error)"=w134, "Message"="WaterInletCloseLDO", "Message Queue"=w138) -> ("error out"=w136:errorcluster, "dup Message Queue"=w135:refnum<queue>)  [unwired: 7 in]
      }
      event "Gas Solenoid Valve Open FVIR": Value Change {
        n51 = event-data() -> ()  [unwired: 1 in, 1 out]
        n52 = call-poly "Enqueue Message.vi"("error in (no error)"=w139, "Message"="GasSolenoidOpenFVIR", "Message Queue"=w143) -> ("error out"=w141:errorcluster, "dup Message Queue"=w140:refnum<queue>)  [unwired: 7 in]
      }
      event "Gas Solenoid Valve Open LDO": Value Change {
        n53 = event-data() -> ()  [unwired: 1 in, 1 out]
        n54 = call-poly "Enqueue Message.vi"("error in (no error)"=w144, "Message"="GasSolenoidOpenLDO", "Message Queue"=w148) -> ("error out"=w146:errorcluster, "dup Message Queue"=w145:refnum<queue>)  [unwired: 7 in]
      }
      event "Gas Solenoid Valve Close FVIR": Value Change {
        n55 = event-data() -> ()  [unwired: 1 in, 1 out]
        n56 = call-poly "Enqueue Message.vi"("error in (no error)"=w149, "Message"="GasSolenoidCloseFVIR", "Message Queue"=w153) -> ("error out"=w151:errorcluster, "dup Message Queue"=w150:refnum<queue>)  [unwired: 7 in]
      }
      event "Gas Solenoid Valve Close LDO": Value Change {
        n57 = event-data() -> ()  [unwired: 1 in, 1 out]
        n58 = call-poly "Enqueue Message.vi"("error in (no error)"=w154, "Message"="GasSolenoidCloseLDO", "Message Queue"=w158) -> ("error out"=w156:errorcluster, "dup Message Queue"=w155:refnum<queue>)  [unwired: 7 in]
      }
      event "Water Flow Intellifaucet DRK375 Open FVIR": Value Change {
        n59 = event-data() -> ()  [unwired: 1 in, 1 out]
        n60 = call-poly "Enqueue Message.vi"("error in (no error)"=w159, "Message"="WaterFlowOpenFVIR", "Message Queue"=w163) -> ("error out"=w161:errorcluster, "dup Message Queue"=w160:refnum<queue>)  [unwired: 7 in]
      }
      event "Water Flow Intellifaucet DRK375 Open LDO": Value Change {
        n61 = event-data() -> ()  [unwired: 1 in, 1 out]
        n62 = call-poly "Enqueue Message.vi"("error in (no error)"=w164, "Message"="WaterFlowStartLDO", "Message Queue"=w173) -> ("error out"=w166:errorcluster, "dup Message Queue"=w171:refnum<queue>)  [unwired: 7 in]
        n63 = for {
          N: 10 -> [_]
          tunnel: w166 -> [w174]
          tunnel: [w174] -> w165
          n64 = Wait Until Next ms Multiple(millisecond multiple=u32 100) -> ()  [unwired: 1 out]
        }
        n65 = call-poly "Enqueue Message.vi"("error in (no error)"=w165, "Message"="WaterFlowStartZeroLDO", "Message Queue"=w171) -> ("error out"=w169:errorcluster, "dup Message Queue"=w170:refnum<queue>)  [unwired: 7 in]
      }
      event "Water Flow Intellifaucet DRK375 Close FVIR": Value Change {
        n66 = event-data() -> ()  [unwired: 1 in, 1 out]
        n67 = call-poly "Enqueue Message.vi"("error in (no error)"=w176, "Message"="WaterFlowCloseFVIR", "Message Queue"=w180) -> ("error out"=w178:errorcluster, "dup Message Queue"=w177:refnum<queue>)  [unwired: 7 in]
      }
      event "Water Flow Intellifaucet DRK375 Close LDO": Value Change {
        n68 = event-data() -> ()  [unwired: 1 in, 1 out]
        n69 = call-poly "Enqueue Message.vi"("error in (no error)"=w181, "Message"="WaterFlowStopLDO", "Message Queue"=w190) -> ("error out"=w183:errorcluster, "dup Message Queue"=w187:refnum<queue>)  [unwired: 7 in]
        n70 = for {
          N: 10 -> [_]
          tunnel: w183 -> [w191]
          tunnel: [w191] -> w182
          n71 = Wait Until Next ms Multiple(millisecond multiple=u32 100) -> ()  [unwired: 1 out]
        }
        n72 = call-poly "Enqueue Message.vi"("error in (no error)"=w182, "Message"="WaterFlowStopZeroLDO", "Message Queue"=w187) -> ("error out"=w188:errorcluster, "dup Message Queue"=w186:refnum<queue>)  [unwired: 7 in]
      }
      event "Water Outlet Flow Proportional Valve EPV-312B Open FVIR": Value Change {
        n73 = event-data() -> ()  [unwired: 1 in, 1 out]
        n74 = call-poly "Enqueue Message.vi"("error in (no error)"=w193, "Message"="WaterFlowPropOpenFVIR", "Message Queue"=w197) -> ("error out"=w195:errorcluster, "dup Message Queue"=w194:refnum<queue>)  [unwired: 7 in]
      }
      event "Water Outlet Flow Proportional Valve EPV-312B Close FVIR": Value Change {
        n75 = event-data() -> ()  [unwired: 1 in, 1 out]
        n76 = call-poly "Enqueue Message.vi"("error in (no error)"=w198, "Message"="WaterFlowPropCloseFVIR", "Message Queue"=w202) -> ("error out"=w200:errorcluster, "dup Message Queue"=w199:refnum<queue>)  [unwired: 7 in]
      }
      event "Oil Spray 0.8 cc/min Open": Value Change {
        n77 = event-data() -> ()  [unwired: 1 in, 1 out]
        n78 = call-poly "Enqueue Message.vi"("error in (no error)"=w203, "Message"="OilSpray08Open", "Message Queue"=w207) -> ("error out"=w205:errorcluster, "dup Message Queue"=w204:refnum<queue>)  [unwired: 7 in]
      }
      event "Oil Spray 0.8 cc/min Close": Value Change {
        n79 = event-data() -> ()  [unwired: 1 in, 1 out]
        n80 = call-poly "Enqueue Message.vi"("error in (no error)"=w208, "Message"="OilSpray08Close", "Message Queue"=w212) -> ("error out"=w210:errorcluster, "dup Message Queue"=w209:refnum<queue>)  [unwired: 7 in]
      }
      event "Oil spray 0.8cc/min - LDO": Value Change {
        n81 = event-data() -> ("NewVal"=w218:bool)  [unwired: 1 in]
        n82 = case shown="False" w218 {
          tunnel: ["OilSpray08Close" ("Message") "OilSpray08Open" ("Message")] -> w214
          frame False {
          }
          frame True {
          }
        }
        n83 = call-poly "Enqueue Message.vi"("error in (no error)"=w213, "Message"=w214, "Message Queue"=w217) -> ("error out"=w216:errorcluster, "dup Message Queue"=w215:refnum<queue>)  [unwired: 7 in]
      }
      event "Oil Spray 1.1 cc/min Open": Value Change {
        n84 = event-data() -> ()  [unwired: 1 in, 1 out]
        n85 = call-poly "Enqueue Message.vi"("error in (no error)"=w221, "Message"="OilSpray11Open", "Message Queue"=w225) -> ("error out"=w223:errorcluster, "dup Message Queue"=w222:refnum<queue>)  [unwired: 7 in]
      }
      event "Oil Spray 1.1 cc/min Close": Value Change {
        n86 = event-data() -> ()  [unwired: 1 in, 1 out]
        n87 = call-poly "Enqueue Message.vi"("error in (no error)"=w226, "Message"="OilSpray11Close", "Message Queue"=w230) -> ("error out"=w228:errorcluster, "dup Message Queue"=w227:refnum<queue>)  [unwired: 7 in]
      }
      event "Oil spray 1.1cc/min - LDO": Value Change {
        n88 = event-data() -> ("NewVal"=w232:bool)  [unwired: 1 in]
        n89 = case shown="True" w232 {
          tunnel: ["OilSpray11Close" ("Message") "OilSpray11Open" ("Message")] -> w236
          frame False {
          }
          frame True {
          }
        }
        n90 = call-poly "Enqueue Message.vi"("error in (no error)"=w231, "Message"=w236, "Message Queue"=w235) -> ("error out"=w233:errorcluster, "dup Message Queue"=w234:refnum<queue>)  [unwired: 7 in]
      }
      event "Oil Spray 1.33 cc/min Open": Value Change {
        n91 = event-data() -> ()  [unwired: 1 in, 1 out]
        n92 = call-poly "Enqueue Message.vi"("error in (no error)"=w239, "Message"="OilSpray133Open", "Message Queue"=w243) -> ("error out"=w241:errorcluster, "dup Message Queue"=w240:refnum<queue>)  [unwired: 7 in]
      }
      event "Oil Spray 1.33 cc/min Close": Value Change {
        n93 = event-data() -> ()  [unwired: 1 in, 1 out]
        n94 = call-poly "Enqueue Message.vi"("error in (no error)"=w244, "Message"="OilSpray133Close", "Message Queue"=w248) -> ("error out"=w246:errorcluster, "dup Message Queue"=w245:refnum<queue>)  [unwired: 7 in]
      }
      event "Oil spray 1.33cc/min - LDO": Value Change {
        n95 = event-data() -> ("NewVal"=w250:bool)  [unwired: 1 in]
        n96 = case shown="True" w250 {
          tunnel: ["OilSpray133Close" ("Message") "OilSpray133Open" ("Message")] -> w254
          frame False {
          }
          frame True {
          }
        }
        n97 = call-poly "Enqueue Message.vi"("error in (no error)"=w249, "Message"=w254, "Message Queue"=w253) -> ("error out"=w251:errorcluster, "dup Message Queue"=w252:refnum<queue>)  [unwired: 7 in]
      }
      event "Heater ON": Value Change {
        n98 = event-data() -> ()  [unwired: 1 in, 1 out]
        n99 = call-poly "Enqueue Message.vi"("error in (no error)"=w257, "Message"="HeaterON", "Message Queue"=w261) -> ("error out"=w259:errorcluster, "dup Message Queue"=w258:refnum<queue>)  [unwired: 7 in]
      }
      event "Heater OFF": Value Change {
        n100 = event-data() -> ()  [unwired: 1 in, 1 out]
        n101 = call-poly "Enqueue Message.vi"("error in (no error)"=w262, "Message"="HeaterOFF", "Message Queue"=w266) -> ("error out"=w264:errorcluster, "dup Message Queue"=w263:refnum<queue>)  [unwired: 7 in]
      }
      event "Send parameters to PLC FVIR": Value Change {
        n102 = event-data() -> ()  [unwired: 1 in, 1 out]
        n103 = call-poly "Enqueue Message.vi"("error in (no error)"=w267, "Message"="SendParamToPLCFVIR", "Message Queue"=w271) -> ("error out"=w269:errorcluster, "dup Message Queue"=w268:refnum<queue>)  [unwired: 7 in]
      }
      event "Send parameters to PLC LDO": Value Change {
        n104 = event-data() -> ()  [unwired: 1 in, 1 out]
        n105 = call-poly "Enqueue Message.vi"("error in (no error)"=w272, "Message"="SendParamToPLCLDO", "Message Queue"=w276) -> ("error out"=w274:errorcluster, "dup Message Queue"=w273:refnum<queue>)  [unwired: 7 in]
      }
      event Panel Close? {
        # "Send the \"Exit\" message if the user closes the panel of the VI. Discard the event so the 'Confirm Quit' message has a chance to run."
        n106 = event-data() -> ()  [unwired: 1 in, 1 out]
        n107 = call-poly "Enqueue Message.vi"("Priority Message? (F)"=TRUE, "error in (no error)"=w277, "Message"="Exit", "Message Queue"=w281) -> ("error out"=w279:errorcluster, "dup Message Queue"=w280:refnum<queue>)  [unwired: 6 in]
        n108 = event-data("Discard?"=TRUE) -> ()  [unwired: 1 in, 1 out]
      }
      event Application Instance Close {
        n109 = event-data() -> ()  [unwired: 1 in, 1 out]
      }
      event User Event {
        w287 = "Exit" ("Exit String")
        # "The Message Handling Loop processed an \"Exit\" message, which fired this event to stop the Event Handling Loop."
        n110 = event-data() -> ()  [unwired: 1 in, 1 out]
        n111 = local write "General status for FVIR"(w287) -> ()
        n112 = local write "General status for LDO"(w287) -> ()
      }
      event Timeout {
        # "The timeout defines how frequencly data should be written to a logfile. When timeout is reach, a request for an additional Modbus read request is send to the Modbus Loop.\nThe shift register is used for checking if the \"Connect\" has been pressed or not."
        n113 = event-data() -> ()  [unwired: 1 in, 1 out]
        n114 = disable-structure shown="Enabled" {
          disable-tunnel: w295 -> [w301 w303]
          disable-tunnel: [w299 w302] -> w294
          disable-tunnel: [w298 w303] -> w292
          disable-tunnel: w291 -> [w297 w302]
          frame Disabled {
            n115 = call-poly "Enqueue Message.vi"("error in (no error)"=w301, "Message"="CheckBeforeWriteDataFVIR", "Message Queue"=w297) -> ("error out"=w298:errorcluster, "dup Message Queue"=w299:refnum<queue>)  [unwired: 7 in]
          }
          frame Enabled {
          }
        }
        n116 = call-poly "Enqueue Message.vi"("error in (no error)"=w292, "Message"="CheckBeforeWriteDataLDO", "Message Queue"=w294) -> ("error out"=w296:errorcluster, "dup Message Queue"=w290:refnum<queue>)  [unwired: 7 in]
      }
      event "Temp (°F)": Value Change {
        n117 = event-data() -> ()  [unwired: 1 in, 1 out]
        n118 = call-poly "Enqueue Message.vi"("Message Data"="Temp (°F)", "Message"="TempChangeDRK375", "Message Queue"=w306) -> ("error out"=w304:errorcluster)  [unwired: 7 in, 1 out]
      }
      event "Valve % Open": Value Change {
        n119 = event-data() -> ()  [unwired: 1 in, 1 out]
        n120 = call-poly "Enqueue Message.vi"("Message Data"="Valve % Open", "Message"="ValveChangeDRK375", "Message Queue"=w311) -> ("error out"=w309:errorcluster)  [unwired: 7 in, 1 out]
      }
      event "Proportioning Valve": Value Change {
        n121 = event-data() -> ()  [unwired: 1 in, 1 out]
        n122 = call-poly "Enqueue Message.vi"("Message Data"="Proportioning Valve", "Message"="ValveChangeEPV", "Message Queue"=w316) -> ("error out"=w314:errorcluster)  [unwired: 7 in, 1 out]
      }
      event "Gas Meter Tare Rate": Value Change {
        n123 = event-data() -> ()  [unwired: 1 in, 1 out]
        n124 = call-poly "Enqueue Message.vi"("Message"="Tare_Flow_LDO", "Message Queue"=w320) -> ("error out"=w319:errorcluster)  [unwired: 8 in, 1 out]
      }
      event "Gas Meter Tare Total": Value Change {
        n125 = event-data() -> ()  [unwired: 1 in, 1 out]
        n126 = call-poly "Enqueue Message.vi"("Message"="Tare_Totalizer_LDO", "Message Queue"=w324) -> ("error out"=w323:errorcluster)  [unwired: 8 in, 1 out]
      }
      event "Reset Flow Meter": Value Change {
        n127 = event-data() -> ()  [unwired: 1 in, 1 out]
        n128 = call-poly "Enqueue Message.vi"("Message"="ResetFlowMeter_ON_LDO", "Message Queue"=w331) -> ("error out"=w328:errorcluster, "dup Message Queue"=w334:refnum<queue>)  [unwired: 8 in]
        n129 = for {
          N: 10 -> [_]
          tunnel: w328 -> [w336]
          tunnel: [w336] -> w327
          n130 = Wait Until Next ms Multiple(millisecond multiple=u32 100) -> ()  [unwired: 1 out]
        }
        n131 = call-poly "Enqueue Message.vi"("error in (no error)"=w327, "Message"="ResetFlowMeter_OFF_LDO", "Message Queue"=w334) -> ("error out"=w330:errorcluster)  [unwired: 7 in, 1 out]
      }
      event "Burner ON": Value Change {
        n132 = event-data() -> ("NewVal"=w341:bool)  [unwired: 1 in, 5 out]
        n133 = case shown="True" w341 {
          tunnel: ["Water_Heater_Status_OFF_LDO" ("Message") "Water_Heater_Status_ON_LDO" ("Message")] -> w338
          frame False {
          }
          frame True {
          }
        }
        n134 = call-poly "Enqueue Message.vi"("Message"=w338, "Message Queue"=w339) -> ("error out"=w340:errorcluster)  [unwired: 8 in, 1 out]
      }
    }
    n135 = call "Error Handler - Event Handling Loop.vi"("error in (no error)"=w43, "Message Queue"=w42) -> ("dup error in"=w44:errorcluster)  [unwired: 8 in, 1 out]
    "Numeric 2" <- w38
  }
  n136 = while {
    tunnel: w19 -> [w367]
    tunnel: w26 -> [w371]
    shift-right: [w365] -> _
    shift-left: w31 -> [w366]
    tunnel: w2 -> [w370]
    tunnel: [w364] -> w36
    tunnel: w24 -> [w361]
    tunnel: w25 -> [w360]
    tunnel: w1 -> [w359]
    shift-right: [w358] -> _
    shift-left: _ -> [w357]
    tunnel: w17 -> [w356]
    tunnel: w14 -> [w355]
    shift-right: [w354] -> _
    shift-left: w15 -> [w353]
    tunnel: w13 -> [w352]
    tunnel: w5 -> [w351]
    shift-right: [w348] -> _
    shift-left: T1 {"Burner ON"=FALSE, "0.8 ml Bool"=FALSE, "1.1 Bool"=FALSE, "1.33 Bool"=FALSE} -> [w349]
    shift-right: [w345] -> _
    shift-left: string[] [] -> [w347]
    i -> [w350]
    stop <- w372 stop-if-true
    # "UI Message Loop"
    n137 = call "Dequeue Message.vi"("error in (no error)"=w370, "Message Queue"=w367) -> ("error out"=w369:errorcluster, "Message Data"=w368:variant, "Message"=w346:string, "dup Message Queue"=w362:refnum<queue>)  [unwired: 6 in]
    n138 = case "Message Cases" shown="\"Initialize\"" w346 {
      selector: w346 -> [_ _ _ _ _ _ _ _ _ _ _ _ _ _ _ _ _ _ _ _ _ _ _ _ _ _ _ _ _ _ _ _ _ _ _ _ _ _ _ _ _ _ _ _ _ _ _ _ _ _ _ _ _ _ _ _ _ _ _ _ _ w1418]
      tunnel: w362 -> [w388 _ _ _ _ w495 w513 _ w552 w576 w664 w676 w688 w700 w708 w728 w748 w768 w792 w804 w816 w828 w840 w852 w864 w876 w888 w900 w912 w924 w936 w948 w960 w972 w984 w996 w1008 w1020 w1027 w1039 w1056 w1068 w1080 w1092 w1104 w1116 w1128 w1140 w1158 w1197 w1209 _ w1310 w1321 w1331 w1345 _ _ _ _ _ _]
      tunnel: w369 -> [w387 w404 w461 w471 w481 w494 w510 w527 w538 w572 w658 w678 w690 w702 w711 w731 w751 w771 w793 w805 w817 w829 w841 w853 w865 w877 w889 w901 w913 w925 w937 w949 w961 w973 w985 w997 w1009 w1021 w1030 w1042 w1057 w1069 w1081 w1093 w1105 w1117 w1129 w1141 w1159 w1198 w1217 w1253 w1313 w1324 w1337 w1350 w1358 w1367 w1374 w1394 w1413 _]
      tunnel: [w379 w404 w462 w472 w482 w490 w516 w527 w547 w569 w663 w673 w685 w696 w714 w734 w754 w774 w795 w807 w819 w831 w843 w855 w867 w879 w891 w903 w915 w927 w939 w951 w963 w975 w987 w999 w1011 w1023 w1029 w1041 w1059 w1071 w1083 w1095 w1107 w1119 w1131 w1143 w1161 w1167 w1218 w1250 w1295 w1319 w1332 w1346 w1357 w1366 w1376 w1405 w1412 w1417] -> w363
      tunnel: [_ _ _ _ _ _ _ _ _ _ _ _ _ _ _ _ _ _ _ _ _ _ _ _ _ _ _ _ _ _ _ _ _ _ _ _ _ _ _ _ _ _ _ _ _ _ _ _ _ _ _ _ _ _ _ _ _ _ _ TRUE _ _] -> w372
      tunnel: w368 -> [_ _ w460 w470 w480 _ _ _ _ _ _ _ _ _ _ _ _ _ _ _ _ _ _ _ _ _ _ _ _ _ _ _ _ _ _ _ _ _ _ _ _ _ _ _ _ _ _ _ _ _ w1216 _ w1312 w1323 w1335 w1349 _ _ w1377 w1402 _ _]
      tunnel: w371 -> [_ _ _ _ _ _ _ _ _ _ _ _ _ _ _ _ _ _ _ _ _ _ _ _ _ _ _ _ _ _ _ _ _ _ _ _ _ _ _ _ _ _ _ _ _ _ _ _ _ _ _ _ _ _ _ _ _ _ _ w1406 _ _]
      tunnel: w366 -> [w400 w406 w456 w466 w478 w491 w506 w529 w549 w578 w668 w680 w692 w704 w709 w729 w749 w769 w790 w802 w814 w826 w838 w850 w862 w874 w886 w898 w910 w922 w934 w946 w958 w970 w982 w994 w1006 w1018 w1036 w1048 w1055 w1067 w1079 w1091 w1103 w1115 w1126 w1138 w1156 w1195 w1214 w1289 w1303 w1326 w1339 w1352 w1361 w1370 w1380 w1404 w1411 w1419]
      tunnel: [w400 w405 w456 w466 w478 w491 w506 w529 w549 w578 w668 w680 w692 w704 w709 w729 w749 w769 w790 w802 w814 w826 w838 w850 w862 w874 w886 w898 w910 w922 w934 w946 w958 w970 w982 w994 w1006 w1018 w1036 w1048 w1055 w1067 w1079 w1091 w1103 w1115 w1126 w1138 w1156 w1195 w1214 w1289 w1303 w1326 w1339 w1352 w1361 w1370 w1380 w1404 w1411 w1419] -> w365
      tunnel: w361 -> [w378 _ _ _ _ _ _ _ w551 w575 w667 w679 w691 w703 w710 w730 w750 w770 w791 w803 w815 w827 w839 w851 w863 w875 w887 w899 w911 w923 w935 w947 w959 w971 w983 w995 w1007 w1019 w1028 w1040 _ _ _ _ _ _ w1127 w1139 w1157 w1196 _ _ _ _ _ _ _ _ _ w1400 _ _]
      tunnel: w360 -> [_ _ _ _ _ w488 w508 _ w550 _ _ _ _ _ _ _ _ _ _ _ _ _ _ _ _ _ _ _ _ _ _ _ _ _ _ _ _ _ _ _ _ _ _ _ _ _ _ _ _ _ _ _ _ _ _ _ _ _ _ w1398 _ _]
      tunnel: w359 -> [_ _ _ _ _ _ _ _ w545 w568 w662 _ _ _ _ _ _ _ _ _ _ _ _ _ _ _ _ _ _ _ _ _ _ _ _ _ _ _ _ _ _ _ _ _ _ _ _ _ _ _ _ _ _ _ _ _ w1356 w1365 _ w1396 _ _]
      tunnel: [FALSE w403 w455 w465 w475 w485 w507 FALSE w532 FALSE w659 w671 w683 w695 w707 w727 w747 w767 w787 w799 w811 w823 w835 w847 w859 w871 w883 w895 w907 w919 w931 w943 w955 w967 w979 w991 w1003 w1015 w1035 w1047 w1052 w1064 w1076 w1088 w1100 w1112 w1123 w1135 w1147 w1180 w1206 w1288 w1308 w1325 w1338 w1351 w1360 w1369 w1373 w1395 w1410 w1416] -> w358
      tunnel: w357 -> [_ w403 w455 w465 w475 w485 w507 _ w532 _ w659 w671 w683 w695 w707 w727 w747 w767 w787 w799 w811 w823 w835 w847 w859 w871 w883 w895 w907 w919 w931 w943 w955 w967 w979 w991 w1003 w1015 w1035 w1047 w1052 w1064 w1076 w1088 w1100 w1112 w1123 w1135 w1147 w1180 w1208 w1288 w1308 w1325 w1338 w1351 w1360 w1369 w1373 w1395 w1410 w1416]
      tunnel: w356 -> [_ _ _ _ _ _ _ _ _ _ _ _ _ _ _ _ _ _ _ _ _ _ _ _ _ _ _ _ _ _ _ _ _ _ _ _ _ _ _ _ w1051 w1063 w1075 w1087 w1099 w1111 _ _ _ _ _ _ _ _ _ _ _ _ _ w1392 _ _]
      tunnel: w355 -> [_ _ _ _ _ _ _ _ _ _ _ _ _ _ _ _ _ _ _ _ _ _ _ _ _ _ _ _ _ _ _ _ _ _ _ _ _ _ _ _ _ _ _ _ _ _ _ _ _ _ _ _ _ _ _ _ _ _ _ w1390 _ _]
      tunnel: w353 -> [w383 w402 w454 w464 w474 w484 w505 w526 w531 w564 w654 w670 w682 w694 w706 w726 w746 w766 w786 w798 w810 w822 w834 w846 w858 w870 w882 w894 w906 w918 w930 w942 w954 w966 w978 w990 w1002 w1014 w1026 w1038 w1050 w1062 w1074 w1086 w1098 w1110 w1122 w1134 w1146 w1175 w1205 w1238 w1293 w1317 w1330 w1344 w1354 w1363 w1372 w1389 w1409 w1415]
      tunnel: [w383 w402 w454 w464 w474 w484 w505 w526 w531 w564 w654 w670 w682 w694 w706 w726 w746 w766 w786 w798 w810 w822 w834 w846 w858 w870 w882 w894 w906 w918 w930 w942 w954 w966 w978 w990 w1002 w1014 w1026 w1038 w1050 w1062 w1074 w1086 w1098 w1110 w1122 w1134 w1146 w1175 w1205 w1237 w1291 w1316 w1329 w1343 w1354 w1363 w1372 w1389 w1409 w1415] -> w354
      tunnel: w352 -> [_ _ _ _ _ _ _ _ _ _ _ _ _ _ _ _ _ _ _ _ _ _ _ _ _ _ _ _ _ _ _ _ _ _ _ _ _ _ _ _ _ _ _ _ _ _ _ _ _ _ _ _ _ _ _ _ _ _ _ w1387 _ _]
      tunnel: w351 -> [_ _ _ _ _ _ _ _ _ _ _ _ _ _ _ _ _ _ _ _ _ _ _ _ _ _ _ _ _ _ _ _ _ _ _ _ _ _ _ _ _ _ _ _ _ _ _ _ _ _ _ _ _ _ _ _ _ _ _ w1383 _ _]
      tunnel: w349 -> [w382 w401 w453 w463 w473 w483 w504 w525 w530 w565 w655 w669 w681 w693 w705 w725 w745 w765 w785 w797 w809 w821 w833 w845 w857 w869 w881 w893 w905 w917 w929 w941 w953 w965 w977 w989 w1001 w1013 w1025 w1037 w1049 w1061 w1073 w1085 w1097 w1109 w1121 w1133 w1145 w1174 w1204 w1245 w1290 w1314 w1327 w1340 w1355 w1364 w1371 w1381 w1408 w1414]
      tunnel: [w382 w401 w453 w463 w473 w483 w504 w525 w530 w565 w655 w669 w681 w693 w705 w725 w745 w765 w785 w797 w809 w821 w833 w845 w857 w869 w881 w893 w905 w917 w929 w941 w953 w965 w977 w989 w1001 w1013 w1025 w1037 w1049 w1061 w1073 w1085 w1097 w1109 w1121 w1133 w1145 w1174 w1204 w1240 w1290 w1314 w1327 w1340 w1355 w1364 w1371 w1381 w1408 w1414] -> w348
      frame "Initialize" {
        w377 = 70.0
        # "Using this flag for checking if the value of the logfile of % Butane is above 1.8. If this is true, this flag will be set to TRUE, if not, it is set to FALSE. This is usefull in the \"StopTestFVIR\" when the value is above 1.8. Because otherwise this will be equal to that the \"STOP\" button will be pressed all the time, and we just want it to be pressed ones."
        # "Reset all values of the HMI"
        # "Initialize - Get configuration settings, then message the UI to initialize, and broadcast the settings to the other message loops."
        n139 = call-poly "Enqueue Message.vi"("error in (no error)"=w387, "Message Data"=u16[] [0, 0, 0, 0, 0, 0, 0, 0] ("Input Registers"), "Message"="DisplayValuesFromPLC", "Message Queue"=w388) -> ("error out"=w386:errorcluster, "dup Message Queue"=w385:refnum<queue>)  [unwired: 6 in]
        n140 = call-poly "Enqueue Message.vi"("error in (no error)"=w386, "Message"="Init UI Refs", "Message Queue"=w385) -> ("error out"=w392:errorcluster, "dup Message Queue"=w391:refnum<queue>)  [unwired: 7 in]
        n141 = call-poly "Enqueue Message.vi"("error in (no error)"=w392, "Message Data"="FVIR Ready..." ("Ready..."), "Message"="Update status - FVIR", "Message Queue"=w391) -> ("error out"=w395:errorcluster, "dup Message Queue"=w396:refnum<queue>)  [unwired: 6 in]
        n142 = call-poly "Enqueue Message.vi"("error in (no error)"=w395, "Message Data"="LDO Ready..." ("Ready..."), "Message"="Update status - LDO", "Message Queue"=w396) -> ("error out"=w380:errorcluster)  [unwired: 6 in, 1 out]
        n143 = call-poly "Enqueue Message.vi"("error in (no error)"=w380, "Message Data"=w377, "Message"="TempChangeDRK375", "Message Queue"=w378) -> ("error out"=w379:errorcluster)  [unwired: 6 in, 1 out]
        n144 = property on="Temp (°F)" class="Slide (strict)"("Value"=w377) -> ()  [unwired: 2 in, 2 out]
      }
      frame "Init UI Refs" {
        # "Init UI Refs - Store control references for UI controls.  Also enable/disable controls appropriately."
        n145 = disable-structure shown="Enabled" {
          disable-tunnel: w406 -> [w451 w452]
          disable-tunnel: [w450 w452] -> w405
          frame Disabled {
            n146 = control-ref of="Start"() -> (w447:refnum<vi>)
            n147 = control-ref of="Stop"() -> (w429:refnum<vi>)
            n148 = control-ref of="Start Test Case FVIR"() -> (w430:refnum<vi>)
            n149 = control-ref of="Stop Test Case FVIR"() -> (w444:refnum<vi>)
            n150 = control-ref of="Water Outlet Valve Open FVIR"() -> (w443:refnum<vi>)
            n151 = control-ref of="Water Outlet Valve Close FVIR"() -> (w442:refnum<vi>)
            n152 = control-ref of="Water Inlet Valve Open FVIR"() -> (w441:refnum<vi>)
            n153 = control-ref of="Water Inlet Valve Close FVIR"() -> (w440:refnum<vi>)
            n154 = control-ref of="Gas Solenoid Valve Open FVIR"() -> (w431:refnum<vi>)
            n155 = control-ref of="Gas Solenoid Valve Close FVIR"() -> (w432:refnum<vi>)
            n156 = control-ref of="Water Flow Intellifaucet DRK375 Open FVIR"() -> (w433:refnum<vi>)
            n157 = control-ref of="Water Flow Intellifaucet DRK375 Close FVIR"() -> (w434:refnum<vi>)
            n158 = control-ref of="Spill can - Go to Home Pos"() -> (w435:refnum<vi>)
            n159 = control-ref of="Spill can - Go to Work Pos"() -> (w436:refnum<vi>)
            n160 = control-ref of="Move mannequin - Go to Home Pos"() -> (w437:refnum<vi>)
            n161 = control-ref of="Move mannequin - Go to Work Pos"() -> (w438:refnum<vi>)
            n162 = control-ref of="Send parameters to PLC FVIR"() -> (w428:refnum<vi>)
            n163 = control-ref of="Water Outlet Flow Proportional Valve EPV-312B Open FVIR"() -> (w427:refnum<vi>)
            n164 = control-ref of="Water Outlet Flow Proportional Valve EPV-312B Close FVIR"() -> (w426:refnum<vi>)
            n165 = control-ref of="Start Test Case LDO"() -> (w425:refnum<vi>)
            n166 = control-ref of="Stop Test Case LDO"() -> (w424:refnum<vi>)
            n167 = control-ref of="Water Outlet Valve Open LDO"() -> (w423:refnum<vi>)
            n168 = control-ref of="Water Outlet Valve Close LDO"() -> (w422:refnum<vi>)
            n169 = control-ref of="Water Inlet Valve Open LDO"() -> (w421:refnum<vi>)
            n170 = control-ref of="Water Inlet Valve Close LDO"() -> (w420:refnum<vi>)
            n171 = control-ref of="Gas Solenoid Valve Open LDO"() -> (w419:refnum<vi>)
            n172 = control-ref of="Gas Solenoid Valve Close LDO"() -> (w418:refnum<vi>)
            n173 = control-ref of="Water Flow Intellifaucet DRK375 Open LDO"() -> (w417:refnum<vi>)
            n174 = control-ref of="Water Flow Intellifaucet DRK375 Close LDO"() -> (w416:refnum<vi>)
            n175 = control-ref of="Oil Spray 0.8 cc/min Open"() -> (w415:refnum<vi>)
            n176 = control-ref of="Oil Spray 0.8 cc/min Close"() -> (w414:refnum<vi>)
            n177 = control-ref of="Oil Spray 1.1 cc/min Open"() -> (w413:refnum<vi>)
            n178 = control-ref of="Oil Spray 1.1 cc/min Close"() -> (w412:refnum<vi>)
            n179 = control-ref of="Oil Spray 1.33 cc/min Open"() -> (w411:refnum<vi>)
            n180 = control-ref of="Oil Spray 1.33 cc/min Close"() -> (w410:refnum<vi>)
            n181 = control-ref of="Heater ON"() -> (w409:refnum<vi>)
            n182 = control-ref of="Heater OFF"() -> (w408:refnum<vi>)
            n183 = control-ref of="Select test case"() -> (w439:refnum<vi>)
            n184 = control-ref of="General status for FVIR"() -> (w407:refnum<vi>)
            n185 = Build Array(w408, w409, w410, w411, w412, w413, w414, w415, w416, w417, w418, w419, w420, w421, w422, w423, w424, w425, w426, w427, w428, w439, w438, w437, w436, w435, w434, w433, w432, w431, w440, w441, w442, w443, w444, w430, w429) -> (w446:refnum<vi>[])
            n186 = Build Array(w447) -> (w445:refnum<vi>[])
            n187 = call "Set Enable State on Multiple Controls.vi"("Enable?"=FALSE, "Controls"=w446) -> ()  [unwired: 10 in]
            n188 = call "Set Enable State on Multiple Controls.vi"("Enable?"=TRUE, "Controls"=w445) -> ()  [unwired: 10 in]
            n189 = Bundle By Name(cluster=w451, "Start Ref"=w447, "Stop Ref"=w429, "Status Ref"=w407, "Start test case FVIR Ref"=w430, "Stop test case FVIR Ref"=w444, "Water Outlet Valve Open FVIR Ref"=w443, "Water Outlet Valve Close FVIR Ref"=w442, "Water Inlet Valve Open FVIR Ref"=w441, "Water Inlet Valve Close FVIR Ref"=w440, "Gas Solenoid Valve Open FVIR Ref"=w431, "Gas Solenoid Valve Close FVIR Ref"=w432, "Water Flow Open FVIR Ref"=w433, "Water Flow Close FVIR Ref"=w434, "Spill can Home pos Ref"=w435, "Spill can Work pos Ref"=w436, "Move Mannequin Home pos Ref"=w437, "Move Mannequin Work pos Ref"=w438, "Listbox Ref"=w439, "Send Param to PLC FVIR Ref"=w428, "Water Flow Prop Open FVIR Ref"=w427, "Water Flow Prop Close FVIR Ref"=w426, "Start test case LDO Ref"=w425, "Stop test case LDO Ref"=w424, "Water Outlet Valve Open LDO Ref"=w423, "Water Outlet Valve Close LDO Ref"=w422, "Water Inlet Valve Open LDO Ref"=w421, "Water Inlet Valve Close LDO Ref"=w420, "Gas Solenoid Valve Open LDO Ref"=w419, "Gas Solenoid Valve Close LDO Ref"=w418, "Water Flow Open LDO Ref"=w417, "Water Flow Close LDO Ref"=w416, "Oil spray 0.8cc/min Open Ref"=w415, "Oil spray 0.8cc/min Close Ref"=w414, "Oil spray 1.1cc/min Open Ref"=w413, "Oil spray 1.1cc/min Close Ref"=w412, "Oil spray 1.33cc/min Open Ref"=w411, "Oil spray 1.33cc/min Close Ref"=w410, "Heater ON Ref"=w409, "Heater OFF Ref"=w408) -> (w450:T11)
          }
          frame Enabled {
          }
        }
      }
      frame "Update status - FVIR" {
        # "Update Status - Convert the message data to a string to display in the Status indicator."
        n190 = Variant To Data(error in=w461, type="", Variant=w460) -> (data=→"General status for FVIR":string, error out=w458:errorcluster)
        n191 = Merge Errors(w458) -> (w462:errorcluster)
      }
      frame "Update status - LDO" {
        # "Update Status - Convert the message data to a string to display in the Status indicator."
        n192 = Variant To Data(error in=w471, type="", Variant=w470) -> (data=→"General status for LDO":string, error out=w468:errorcluster)
        n193 = Merge Errors(w468) -> (w472:errorcluster)
      }
      frame "ShowLabViewLifeBit" {
        # "Update Status - Convert the message data to a string to display in the Status indicator."
        n194 = Variant To Data(error in=w481, type=TRUE, Variant=w480) -> (data=→"Labview lifebit":bool, error out=w479:errorcluster)
        n195 = Merge Errors(w479) -> (w482:errorcluster)
      }
      frame "Start" {
        # "Note: So right now, I am writing to the HMI that we only read the log file. \nHowever the acqusition and logging from the original template does also happens, which needs to be \ncleaned up later."
        # "Start - Enable/Disable buttons appropriately for an acquisition that has started, and update status display."
        n196 = disable-structure shown="Disabled" {
          disable-tunnel: w491 -> [w503 _]
          frame Disabled {
            # "Enable: Stop\nDisable: Start, Exit, Settings"
            n197 = Unbundle By Name(w503) -> ("Stop Ref"=w498:refnum<vi>, "Start Ref"=w497:refnum<vi>, "Exit Ref"=w496:refnum<vi>)
            n198 = Build Array(w497, w496) -> (w501:refnum<vi>[])
            n199 = Build Array(w498) -> (w500:refnum<vi>[])
            n200 = call "Set Enable State on Multiple Controls.vi"("Enable?"=FALSE, "Controls"=w501) -> ()  [unwired: 10 in]
            n201 = call "Set Enable State on Multiple Controls.vi"("Enable?"=TRUE, "Controls"=w500) -> ()  [unwired: 10 in]
          }
          frame Enabled {
          }
        }
        n202 = call-poly "Enqueue Message.vi"("error in (no error)"=w494, "Message Data"="Starting to read log file..." ("Acquiring and Logging..."), "Message"="Update Status - FVIR", "Message Queue"=w495) -> ("error out"=w487:errorcluster)  [unwired: 6 in, 1 out]
        n203 = call-poly "Enqueue Message.vi"("error in (no error)"=w487, "Message Data"="Path to local logfile", "Message"="Start", "Message Queue"=w488) -> ("error out"=w490:errorcluster)  [unwired: 6 in, 1 out]
      }
      frame "Stop" {
        # "Stop - Enable/Disable buttons appropriately for an acquisition that has stopped, and update status display."
        n204 = disable-structure shown="Disabled" {
          disable-tunnel: w506 -> [w517 _]
          frame Disabled {
            n205 = Unbundle By Name(w517) -> ("Stop Ref"=w523:refnum<vi>, "Start Ref"=w521:refnum<vi>, "Exit Ref"=w520:refnum<vi>)
            n206 = Build Array(w523) -> (w519:refnum<vi>[])
            n207 = Build Array(w521, w520) -> (w518:refnum<vi>[])
            n208 = call "Set Enable State on Multiple Controls.vi"("Enable?"=FALSE, "Controls"=w519) -> ()  [unwired: 10 in]
            n209 = call "Set Enable State on Multiple Controls.vi"("Enable?"=TRUE, "Controls"=w518) -> ()  [unwired: 10 in]
          }
          frame Enabled {
          }
        }
        n210 = call-poly "Enqueue Message.vi"("error in (no error)"=w510, "Message Data"="Stopping to read log file..." ("Acquiring and Logging..."), "Message"="Update Status - FVIR", "Message Queue"=w513) -> ("error out"=w509:errorcluster)  [unwired: 6 in, 1 out]
        n211 = call-poly "Enqueue Message.vi"("error in (no error)"=w509, "Message"="Stop", "Message Queue"=w508) -> ("error out"=w515:errorcluster)  [unwired: 7 in, 1 out]
        n212 = Merge Errors(w515) -> (w516:errorcluster)
      }
      frame "Connect" {
        # "Start - Enable/Disable buttons appropriately for an acquisition that has started, and update status display."
      }
      frame "Disconnect" {
        w546 = "Disconnect" ("Message")
        # "Sending an \"init\" so \nthat all the buttons gets back to disabled"
        # "Enable: Connect\nDisable: Disconnect, Move mannequin, Spill Can, Water Outlet Valve, Exit"
        # "Message Modbus Message and RedDataFile loops to disconnect."
        # "Start - Enable/Disable buttons appropriately for an acquisition that has started, and update status display."
        n213 = disable-structure shown="Disabled" {
          disable-tunnel: w549 -> [w558 _]
          frame Disabled {
            n214 = Unbundle By Name(w558) -> ("Disconnect Ref"=w557:refnum<vi>, "Connect Ref"=w555:refnum<vi>, "Exit Ref"=w554:refnum<vi>)
            n215 = Build Array(w557) -> (w560:refnum<vi>[])
            n216 = Build Array(w555, w554) -> (w553:refnum<vi>[])
            n217 = call "Set Enable State on Multiple Controls.vi"("Enable?"=FALSE, "Controls"=w560) -> ()  [unwired: 10 in]
            n218 = call "Set Enable State on Multiple Controls.vi"("Enable?"=TRUE, "Controls"=w553) -> ()  [unwired: 10 in]
          }
          frame Enabled {
          }
        }
        n219 = call-poly "Enqueue Message.vi"("error in (no error)"=w538, "Message Data"="Disconnecting with Modbus TCP/IP..." ("Acquiring and Logging..."), "Message"="Update Status - FVIR", "Message Queue"=w552) -> ("error out"=w537:errorcluster, "dup Message Queue"=w542:refnum<queue>)  [unwired: 6 in]
        n220 = call-poly "Enqueue Message.vi"("error in (no error)"=w537, "Message Data"="Disconnecting with Modbus TCP/IP..." ("Acquiring and Logging..."), "Message"="Update Status - LDO", "Message Queue"=w542) -> ("error out"=w541:errorcluster, "dup Message Queue"=w540:refnum<queue>)  [unwired: 6 in]
        n221 = call-poly "Enqueue Message.vi"("error in (no error)"=w541, "Message"="Init UI Refs", "Message Queue"=w540) -> ("error out"=w536:errorcluster)  [unwired: 7 in, 1 out]
        n222 = call-poly "Enqueue Message.vi"("error in (no error)"=w536, "Message"=w546, "Message Queue"=w551) -> ("error out"=w535:errorcluster)  [unwired: 7 in, 1 out]
        n223 = call-poly "Enqueue Message.vi"("error in (no error)"=w535, "Message"=w546, "Message Queue"=w550) -> ("error out"=w534:errorcluster)  [unwired: 7 in, 1 out]
        n224 = call-poly "Enqueue Message.vi"("error in (no error)"=w534, "Message"=w546, "Message Queue"=w545) -> ("error out"=w547:errorcluster)  [unwired: 7 in, 1 out]
      }
      frame "StartTestCaseFVIR" {
        # "When the operator starts a test, the information about \nthe test is passed to the Writing DataFile Loop"
        # "Indicate that now a FVIR test is active"
        # "Start - Enable/Disable buttons appropriately for an acquisition that has started, and update status display."
        n225 = call-poly "Enqueue Message.vi"("error in (no error)"=w572, "Message"="StartTestFVIR", "Message Queue"=w575) -> ("error out"=w571:errorcluster, "dup Message Queue"=w574:refnum<queue>)  [unwired: 7 in]
        n226 = case shown="0, Default" "Select test case" {
          tunnel: w576 -> [w585 w594 w603 w612 w621 w630 w639 w648]
          tunnel: w571 -> [w584 w593 w602 w611 w620 w629 w638 w647]
          tunnel: w574 -> [w582 w591 w600 w609 w618 w627 w636 w645]
          tunnel: [w581 w590 w599 w608 w617 w626 w635 w644] -> w570
          tunnel: ["FV_case_1_Winter" ("Acquiring and Logging...") "FV_ case _1_Summer" ("Acquiring and Logging...") "FV_case _2_Winter" ("Acquiring and Logging...") "FV_case_2_Summer" ("Acquiring and Logging...") "FV_case_3_Winter" ("Acquiring and Logging...") "FV_case_3_Summer" ("Acquiring and Logging...") "FV_case_4_Winter" ("Acquiring and Logging...") "FV_case _4_Summer" ("Acquiring and Logging...")] -> w563
          frame 0, Default {
            n227 = call-poly "Enqueue Message.vi"("error in (no error)"=w584, "Message Data"="Test case #1 - Winter has started ..." ("Acquiring and Logging..."), "Message"="Update Status - FVIR", "Message Queue"=w585) -> ("error out"=w583:errorcluster)  [unwired: 6 in, 1 out]
            n228 = call-poly "Enqueue Message.vi"("error in (no error)"=w583, "Message"="TestCase1Winter", "Message Queue"=w582) -> ("error out"=w581:errorcluster)  [unwired: 7 in, 1 out]
          }
          frame 1 {
            n229 = call-poly "Enqueue Message.vi"("error in (no error)"=w593, "Message Data"="Test case #1 - Summer has started ..." ("Acquiring and Logging..."), "Message"="Update Status - FVIR", "Message Queue"=w594) -> ("error out"=w592:errorcluster)  [unwired: 6 in, 1 out]
            n230 = call-poly "Enqueue Message.vi"("error in (no error)"=w592, "Message"="TestCase1Summer", "Message Queue"=w591) -> ("error out"=w590:errorcluster)  [unwired: 7 in, 1 out]
          }
          frame 2 {
            n231 = call-poly "Enqueue Message.vi"("error in (no error)"=w602, "Message Data"="Test case #2 - Winter has started ..." ("Acquiring and Logging..."), "Message"="Update Status - FVIR", "Message Queue"=w603) -> ("error out"=w601:errorcluster)  [unwired: 6 in, 1 out]
            n232 = call-poly "Enqueue Message.vi"("error in (no error)"=w601, "Message"="TestCase2Winter", "Message Queue"=w600) -> ("error out"=w599:errorcluster)  [unwired: 7 in, 1 out]
          }
          frame 3 {
            n233 = call-poly "Enqueue Message.vi"("error in (no error)"=w611, "Message Data"="Test case #2 - Summer has started ..." ("Acquiring and Logging..."), "Message"="Update Status - FVIR", "Message Queue"=w612) -> ("error out"=w610:errorcluster)  [unwired: 6 in, 1 out]
            n234 = call-poly "Enqueue Message.vi"("error in (no error)"=w610, "Message"="TestCase2Summer", "Message Queue"=w609) -> ("error out"=w608:errorcluster)  [unwired: 7 in, 1 out]
          }
          frame 4 {
            n235 = call-poly "Enqueue Message.vi"("error in (no error)"=w620, "Message Data"="Test case #3 - Winter has started ..." ("Acquiring and Logging..."), "Message"="Update Status - FVIR", "Message Queue"=w621) -> ("error out"=w619:errorcluster)  [unwired: 6 in, 1 out]
            n236 = call-poly "Enqueue Message.vi"("error in (no error)"=w619, "Message"="TestCase3Winter", "Message Queue"=w618) -> ("error out"=w617:errorcluster)  [unwired: 7 in, 1 out]
          }
          frame 5 {
            n237 = call-poly "Enqueue Message.vi"("error in (no error)"=w629, "Message Data"="Test case #3 - Summer has started ..." ("Acquiring and Logging..."), "Message"="Update Status - FVIR", "Message Queue"=w630) -> ("error out"=w628:errorcluster)  [unwired: 6 in, 1 out]
            n238 = call-poly "Enqueue Message.vi"("error in (no error)"=w628, "Message"="TestCase3Summer", "Message Queue"=w627) -> ("error out"=w626:errorcluster)  [unwired: 7 in, 1 out]
          }
          frame 6 {
            n239 = call-poly "Enqueue Message.vi"("error in (no error)"=w638, "Message Data"="Test case #4 - Winter has started ..." ("Acquiring and Logging..."), "Message"="Update Status - FVIR", "Message Queue"=w639) -> ("error out"=w637:errorcluster)  [unwired: 6 in, 1 out]
            n240 = call-poly "Enqueue Message.vi"("error in (no error)"=w637, "Message"="TestCase4Winter", "Message Queue"=w636) -> ("error out"=w635:errorcluster)  [unwired: 7 in, 1 out]
          }
          frame 7 {
            n241 = call-poly "Enqueue Message.vi"("error in (no error)"=w647, "Message Data"="Test case #4 - Summer has started ..." ("Acquiring and Logging..."), "Message"="Update Status - FVIR", "Message Queue"=w648) -> ("error out"=w646:errorcluster)  [unwired: 6 in, 1 out]
            n242 = call-poly "Enqueue Message.vi"("error in (no error)"=w646, "Message"="TestCase4Summer", "Message Queue"=w645) -> ("error out"=w644:errorcluster)  [unwired: 7 in, 1 out]
          }
        }
        n243 = Bundle By Name(cluster=w564, "PLC Data Out.Data to Save.Test Case - FVIR"=w563) -> (w562:T2)
        n244 = Unbundle By Name(w562) -> ("PLC Data Out"=w561:T3)
        n245 = call-poly "Enqueue Message.vi"("error in (no error)"=w570, "Message Data"=w561, "Message"="InsertTextIntoDataFileNameFVIR", "Message Queue"=w568) -> ("error out"=w569:errorcluster)  [unwired: 6 in, 1 out]
      }
      frame "StartTestCaseLDO" {
        # "Indicate that now a LDO test is active"
        # "Start - Enable/Disable buttons appropriately for an acquisition that has started, and update status display."
        n246 = call-poly "Enqueue Message.vi"("error in (no error)"=w658, "Message Data"="LDO test has started..." ("Acquiring and Logging..."), "Message"="Update Status - LDO", "Message Queue"=w664) -> ("error out"=w657:errorcluster)  [unwired: 6 in, 1 out]
        n247 = call-poly "Enqueue Message.vi"("error in (no error)"=w657, "Message"="StartTestLDO", "Message Queue"=w667) -> ("error out"=w656:errorcluster)  [unwired: 7 in, 1 out]
        n248 = Bundle By Name(cluster=w654, "PLC Data Out.Data to Save.Test Case - LDO"="LDO_test" ("Acquiring and Logging...")) -> (w652:T2)
        n249 = Unbundle By Name(w652) -> ("PLC Data Out"=w651:T3)
        n250 = call-poly "Enqueue Message.vi"("error in (no error)"=w656, "Message Data"=w651, "Message"="InsertTextIntoDataFileNameLDO", "Message Queue"=w662) -> ("error out"=w663:errorcluster)  [unwired: 6 in, 1 out]
      }
      frame "StopTestCaseFVIR" {
        # "Start - Enable/Disable buttons appropriately for an acquisition that has started, and update status display."
        n251 = call-poly "Enqueue Message.vi"("error in (no error)"=w678, "Message"="StopTestFVIR", "Message Queue"=w679) -> ("error out"=w675:errorcluster)  [unwired: 7 in, 1 out]
        n252 = call-poly "Enqueue Message.vi"("error in (no error)"=w675, "Message Data"="Current FVIR test has stopped ..." ("Acquiring and Logging..."), "Message"="Update Status - FVIR", "Message Queue"=w676) -> ("error out"=w673:errorcluster)  [unwired: 6 in, 1 out]
      }
      frame "StopTestCaseFVIRLogFile" {
        # "Start - Enable/Disable buttons appropriately for an acquisition that has started, and update status display."
        n253 = call-poly "Enqueue Message.vi"("error in (no error)"=w690, "Message"="StopTestFVIR", "Message Queue"=w691) -> ("error out"=w687:errorcluster)  [unwired: 7 in, 1 out]
        n254 = call-poly "Enqueue Message.vi"("error in (no error)"=w687, "Message Data"="Current FVIR test has stopped ..." ("Acquiring and Logging..."), "Message"="Update Status - FVIR", "Message Queue"=w688) -> ("error out"=w685:errorcluster)  [unwired: 6 in, 1 out]
      }
      frame "StopTestCaseLDO" {
        # "Start - Enable/Disable buttons appropriately for an acquisition that has started, and update status display."
        n255 = call-poly "Enqueue Message.vi"("error in (no error)"=w702, "Message"="StopTestLDO", "Message Queue"=w703) -> ("error out"=w699:errorcluster)  [unwired: 7 in, 1 out]
        n256 = call-poly "Enqueue Message.vi"("error in (no error)"=w699, "Message Data"="Current LDO test has stopped ..." ("Acquiring and Logging..."), "Message"="Update Status - LDO", "Message Queue"=w700) -> ("error out"=w696:errorcluster)  [unwired: 6 in, 1 out]
      }
      frame "MannequinHomePos" {
        # "Start - Enable/Disable buttons appropriately for an acquisition that has started, and update status display."
        n257 = disable-structure shown="Disabled" {
          disable-tunnel: w709 -> [w717 _]
          frame Disabled {
            n258 = Unbundle By Name(w717) -> ("Stop Ref"=w722:refnum<vi>, "Start Ref"=w721:refnum<vi>, "Exit Ref"=w720:refnum<vi>)
            n259 = Build Array(w722) -> (w723:refnum<vi>[])
            n260 = Build Array(w721, w720) -> (w724:refnum<vi>[])
            n261 = call "Set Enable State on Multiple Controls.vi"("Enable?"=TRUE, "Controls"=w723) -> ()  [unwired: 10 in]
            n262 = call "Set Enable State on Multiple Controls.vi"("Enable?"=FALSE, "Controls"=w724) -> ()  [unwired: 10 in]
          }
          frame Enabled {
          }
        }
        n263 = call-poly "Enqueue Message.vi"("error in (no error)"=w711, "Message Data"="Operator clicked on: Move mannequin to Home Pos" ("Acquiring and Logging..."), "Message"="Update Status - FVIR", "Message Queue"=w708) -> ("error out"=w712:errorcluster)  [unwired: 6 in, 1 out]
        n264 = call-poly "Enqueue Message.vi"("error in (no error)"=w712, "Message"="MannequinGoToHomePos", "Message Queue"=w710) -> ("error out"=w714:errorcluster)  [unwired: 7 in, 1 out]
      }
      frame "MannequinWorkPos" {
        # "Start - Enable/Disable buttons appropriately for an acquisition that has started, and update status display."
        n265 = disable-structure shown="Disabled" {
          disable-tunnel: w729 -> [w737 _]
          frame Disabled {
            n266 = Unbundle By Name(w737) -> ("Stop Ref"=w742:refnum<vi>, "Start Ref"=w741:refnum<vi>, "Exit Ref"=w740:refnum<vi>)
            n267 = Build Array(w742) -> (w743:refnum<vi>[])
            n268 = Build Array(w741, w740) -> (w744:refnum<vi>[])
            n269 = call "Set Enable State on Multiple Controls.vi"("Enable?"=TRUE, "Controls"=w743) -> ()  [unwired: 10 in]
            n270 = call "Set Enable State on Multiple Controls.vi"("Enable?"=FALSE, "Controls"=w744) -> ()  [unwired: 10 in]
          }
          frame Enabled {
          }
        }
        n271 = call-poly "Enqueue Message.vi"("error in (no error)"=w731, "Message Data"="Operator clicked on: Move mannequin to Work Pos" ("Acquiring and Logging..."), "Message"="Update Status - FVIR", "Message Queue"=w728) -> ("error out"=w732:errorcluster)  [unwired: 6 in, 1 out]
        n272 = call-poly "Enqueue Message.vi"("error in (no error)"=w732, "Message"="MannequinGoToWorkPos", "Message Queue"=w730) -> ("error out"=w734:errorcluster)  [unwired: 7 in, 1 out]
      }
      frame "SpillCanHomePos" {
        # "Start - Enable/Disable buttons appropriately for an acquisition that has started, and update status display."
        n273 = disable-structure shown="Disabled" {
          disable-tunnel: w749 -> [w757 _]
          frame Disabled {
            n274 = Unbundle By Name(w757) -> ("Stop Ref"=w762:refnum<vi>, "Start Ref"=w761:refnum<vi>, "Exit Ref"=w760:refnum<vi>)
            n275 = Build Array(w762) -> (w763:refnum<vi>[])
            n276 = Build Array(w761, w760) -> (w764:refnum<vi>[])
            n277 = call "Set Enable State on Multiple Controls.vi"("Enable?"=TRUE, "Controls"=w763) -> ()  [unwired: 10 in]
            n278 = call "Set Enable State on Multiple Controls.vi"("Enable?"=FALSE, "Controls"=w764) -> ()  [unwired: 10 in]
          }
          frame Enabled {
          }
        }
        n279 = call-poly "Enqueue Message.vi"("error in (no error)"=w751, "Message Data"="Operator clicked on: Move gasoline can to Home Pos" ("Acquiring and Logging..."), "Message"="Update Status - FVIR", "Message Queue"=w748) -> ("error out"=w752:errorcluster)  [unwired: 6 in, 1 out]
        n280 = call-poly "Enqueue Message.vi"("error in (no error)"=w752, "Message"="SpillCanGoToHomePos", "Message Queue"=w750) -> ("error out"=w754:errorcluster)  [unwired: 7 in, 1 out]
      }
      frame "SpillCanWorkPos" {
        # "Start - Enable/Disable buttons appropriately for an acquisition that has started, and update status display."
        n281 = disable-structure shown="Disabled" {
          disable-tunnel: w769 -> [w777 _]
          frame Disabled {
            n282 = Unbundle By Name(w777) -> ("Stop Ref"=w782:refnum<vi>, "Start Ref"=w781:refnum<vi>, "Exit Ref"=w780:refnum<vi>)
            n283 = Build Array(w782) -> (w783:refnum<vi>[])
            n284 = Build Array(w781, w780) -> (w784:refnum<vi>[])
            n285 = call "Set Enable State on Multiple Controls.vi"("Enable?"=TRUE, "Controls"=w783) -> ()  [unwired: 10 in]
            n286 = call "Set Enable State on Multiple Controls.vi"("Enable?"=FALSE, "Controls"=w784) -> ()  [unwired: 10 in]
          }
          frame Enabled {
          }
        }
        n287 = call-poly "Enqueue Message.vi"("error in (no error)"=w771, "Message Data"="Operator clicked on: Move gasoline can to Work Pos" ("Acquiring and Logging..."), "Message"="Update Status - FVIR", "Message Queue"=w768) -> ("error out"=w772:errorcluster)  [unwired: 6 in, 1 out]
        n288 = call-poly "Enqueue Message.vi"("error in (no error)"=w772, "Message"="SpillCanGoToWorkPos", "Message Queue"=w770) -> ("error out"=w774:errorcluster)  [unwired: 7 in, 1 out]
      }
      frame "WaterOutletOpenFVIR" {
        # "Start - Enable/Disable buttons appropriately for an acquisition that has started, and update status display."
        n289 = call-poly "Enqueue Message.vi"("error in (no error)"=w793, "Message Data"="Operator clicked on: Water Outlet Valve Open FVIR" ("Acquiring and Logging..."), "Message"="Update Status - FVIR", "Message Queue"=w792) -> ("error out"=w794:errorcluster)  [unwired: 6 in, 1 out]
        n290 = call-poly "Enqueue Message.vi"("error in (no error)"=w794, "Message"="WaterOutletOpenFVIR", "Message Queue"=w791) -> ("error out"=w795:errorcluster)  [unwired: 7 in, 1 out]
      }
      frame "WaterOutletOpenLDO" {
        # "Start - Enable/Disable buttons appropriately for an acquisition that has started, and update status display."
        n291 = call-poly "Enqueue Message.vi"("error in (no error)"=w805, "Message Data"="Operator clicked on: Water Outlet Valve Open LDO" ("Acquiring and Logging..."), "Message"="Update Status - LDO", "Message Queue"=w804) -> ("error out"=w806:errorcluster)  [unwired: 6 in, 1 out]
        n292 = call-poly "Enqueue Message.vi"("error in (no error)"=w806, "Message"="WaterOutletOpenLDO", "Message Queue"=w803) -> ("error out"=w807:errorcluster)  [unwired: 7 in, 1 out]
      }
      frame "WaterOutletCloseFVIR" {
        # "Start - Enable/Disable buttons appropriately for an acquisition that has started, and update status display."
        n293 = call-poly "Enqueue Message.vi"("error in (no error)"=w817, "Message Data"="Operator clicked on: Water Outlet Valve Close FVIR" ("Acquiring and Logging..."), "Message"="Update Status - FVIR", "Message Queue"=w816) -> ("error out"=w818:errorcluster)  [unwired: 6 in, 1 out]
        n294 = call-poly "Enqueue Message.vi"("error in (no error)"=w818, "Message"="WaterOutletCloseFVIR", "Message Queue"=w815) -> ("error out"=w819:errorcluster)  [unwired: 7 in, 1 out]
      }
      frame "WaterOutletCloseLDO" {
        # "Start - Enable/Disable buttons appropriately for an acquisition that has started, and update status display."
        n295 = call-poly "Enqueue Message.vi"("error in (no error)"=w829, "Message Data"="Operator clicked on: Water Outlet Valve Close LDO" ("Acquiring and Logging..."), "Message"="Update Status - LDO", "Message Queue"=w828) -> ("error out"=w830:errorcluster)  [unwired: 6 in, 1 out]
        n296 = call-poly "Enqueue Message.vi"("error in (no error)"=w830, "Message"="WaterOutletCloseLDO", "Message Queue"=w827) -> ("error out"=w831:errorcluster)  [unwired: 7 in, 1 out]
      }
      frame "WaterInletOpenFVIR" {
        # "Start - Enable/Disable buttons appropriately for an acquisition that has started, and update status display."
        n297 = call-poly "Enqueue Message.vi"("error in (no error)"=w841, "Message Data"="Operator clicked on: Water Inlet Valve Open FVIR" ("Acquiring and Logging..."), "Message"="Update Status - FVIR", "Message Queue"=w840) -> ("error out"=w842:errorcluster)  [unwired: 6 in, 1 out]
        n298 = call-poly "Enqueue Message.vi"("error in (no error)"=w842, "Message"="WaterInletOpenFVIR", "Message Queue"=w839) -> ("error out"=w843:errorcluster)  [unwired: 7 in, 1 out]
      }
      frame "WaterInletOpenLDO" {
        # "Start - Enable/Disable buttons appropriately for an acquisition that has started, and update status display."
        n299 = call-poly "Enqueue Message.vi"("error in (no error)"=w853, "Message Data"="Operator clicked on: Water Inlet Valve Open LDO" ("Acquiring and Logging..."), "Message"="Update Status - LDO", "Message Queue"=w852) -> ("error out"=w854:errorcluster)  [unwired: 6 in, 1 out]
        n300 = call-poly "Enqueue Message.vi"("error in (no error)"=w854, "Message"="WaterInletOpenLDO", "Message Queue"=w851) -> ("error out"=w855:errorcluster)  [unwired: 7 in, 1 out]
      }
      frame "WaterInletCloseFVIR" {
        # "Start - Enable/Disable buttons appropriately for an acquisition that has started, and update status display."
        n301 = call-poly "Enqueue Message.vi"("error in (no error)"=w865, "Message Data"="Operator clicked on: Water Inlet Valve Close FVIR" ("Acquiring and Logging..."), "Message"="Update Status - FVIR", "Message Queue"=w864) -> ("error out"=w866:errorcluster)  [unwired: 6 in, 1 out]
        n302 = call-poly "Enqueue Message.vi"("error in (no error)"=w866, "Message"="WaterInletCloseFVIR", "Message Queue"=w863) -> ("error out"=w867:errorcluster)  [unwired: 7 in, 1 out]
      }
      frame "WaterInletCloseLDO" {
        # "Start - Enable/Disable buttons appropriately for an acquisition that has started, and update status display."
        n303 = call-poly "Enqueue Message.vi"("error in (no error)"=w877, "Message Data"="Operator clicked on: Water Inlet Valve Close LDO" ("Acquiring and Logging..."), "Message"="Update Status - LDO", "Message Queue"=w876) -> ("error out"=w878:errorcluster)  [unwired: 6 in, 1 out]
        n304 = call-poly "Enqueue Message.vi"("error in (no error)"=w878, "Message"="WaterInletCloseLDO", "Message Queue"=w875) -> ("error out"=w879:errorcluster)  [unwired: 7 in, 1 out]
      }
      frame "GasSolenoidOpenFVIR" {
        # "Start - Enable/Disable buttons appropriately for an acquisition that has started, and update status display."
        n305 = call-poly "Enqueue Message.vi"("error in (no error)"=w889, "Message Data"="Operator clicked on: Gas Solenoid Valve Open FVIR" ("Acquiring and Logging..."), "Message"="Update Status - FVIR", "Message Queue"=w888) -> ("error out"=w890:errorcluster)  [unwired: 6 in, 1 out]
        n306 = call-poly "Enqueue Message.vi"("error in (no error)"=w890, "Message"="GasSolenoidOpenFVIR", "Message Queue"=w887) -> ("error out"=w891:errorcluster)  [unwired: 7 in, 1 out]
      }
      frame "GasSolenoidOpenLDO" {
        # "Start - Enable/Disable buttons appropriately for an acquisition that has started, and update status display."
        n307 = call-poly "Enqueue Message.vi"("error in (no error)"=w901, "Message Data"="Operator clicked on: Gas Solenoid Valve Open LDO" ("Acquiring and Logging..."), "Message"="Update Status - LDO", "Message Queue"=w900) -> ("error out"=w902:errorcluster)  [unwired: 6 in, 1 out]
        n308 = call-poly "Enqueue Message.vi"("error in (no error)"=w902, "Message"="GasSolenoidOpenLDO", "Message Queue"=w899) -> ("error out"=w903:errorcluster)  [unwired: 7 in, 1 out]
      }
      frame "GasSolenoidCloseFVIR" {
        # "Start - Enable/Disable buttons appropriately for an acquisition that has started, and update status display."
        n309 = call-poly "Enqueue Message.vi"("error in (no error)"=w913, "Message Data"="Operator clicked on: Gas Solenoid Valve Close FVIR" ("Acquiring and Logging..."), "Message"="Update Status - FVIR", "Message Queue"=w912) -> ("error out"=w914:errorcluster)  [unwired: 6 in, 1 out]
        n310 = call-poly "Enqueue Message.vi"("error in (no error)"=w914, "Message"="GasSolenoidCloseFVIR", "Message Queue"=w911) -> ("error out"=w915:errorcluster)  [unwired: 7 in, 1 out]
      }
      frame "GasSolenoidCloseLDO" {
        # "Start - Enable/Disable buttons appropriately for an acquisition that has started, and update status display."
        n311 = call-poly "Enqueue Message.vi"("error in (no error)"=w925, "Message Data"="Operator clicked on: Gas Solenoid Valve Close LDO" ("Acquiring and Logging..."), "Message"="Update Status - LDO", "Message Queue"=w924) -> ("error out"=w926:errorcluster)  [unwired: 6 in, 1 out]
        n312 = call-poly "Enqueue Message.vi"("error in (no error)"=w926, "Message"="GasSolenoidCloseLDO", "Message Queue"=w923) -> ("error out"=w927:errorcluster)  [unwired: 7 in, 1 out]
      }
      frame "WaterFlowOpenFVIR" {
        # "Start - Enable/Disable buttons appropriately for an acquisition that has started, and update status display."
        n313 = call-poly "Enqueue Message.vi"("error in (no error)"=w937, "Message Data"="Operator clicked on: Water Flow Intellifaucet DRK375 Open FVIR" ("Acquiring and Logging..."), "Message"="Update Status - FVIR", "Message Queue"=w936) -> ("error out"=w938:errorcluster)  [unwired: 6 in, 1 out]
        n314 = call-poly "Enqueue Message.vi"("error in (no error)"=w938, "Message"="WaterFlowOpenFVIR", "Message Queue"=w935) -> ("error out"=w939:errorcluster)  [unwired: 7 in, 1 out]
      }
      frame "WaterFlowStartLDO" {
        # "Start - Enable/Disable buttons appropriately for an acquisition that has started, and update status display."
        n315 = call-poly "Enqueue Message.vi"("error in (no error)"=w949, "Message Data"="Operator clicked on: Water Flow Intellifaucet DRK375 Start" ("Acquiring and Logging..."), "Message"="Update Status - LDO", "Message Queue"=w948) -> ("error out"=w950:errorcluster)  [unwired: 6 in, 1 out]
        n316 = call-poly "Enqueue Message.vi"("error in (no error)"=w950, "Message"="WaterFlowStartLDO", "Message Queue"=w947) -> ("error out"=w951:errorcluster)  [unwired: 7 in, 1 out]
      }
      frame "WaterFlowCloseFVIR" {
        # "Start - Enable/Disable buttons appropriately for an acquisition that has started, and update status display."
        n317 = call-poly "Enqueue Message.vi"("error in (no error)"=w961, "Message Data"="Operator clicked on: Water Flow Intellifaucet DRK375 Close FVIR" ("Acquiring and Logging..."), "Message"="Update Status - FVIR", "Message Queue"=w960) -> ("error out"=w962:errorcluster)  [unwired: 6 in, 1 out]
        n318 = call-poly "Enqueue Message.vi"("error in (no error)"=w962, "Message"="WaterFlowCloseFVIR", "Message Queue"=w959) -> ("error out"=w963:errorcluster)  [unwired: 7 in, 1 out]
      }
      frame "WaterFlowStartZeroLDO" {
        # "Start - Enable/Disable buttons appropriately for an acquisition that has started, and update status display."
        n319 = call-poly "Enqueue Message.vi"("error in (no error)"=w973, "Message Data"="Operator clicked on: Water Flow Intellifaucet DRK375 Start" ("Acquiring and Logging..."), "Message"="Update Status - LDO", "Message Queue"=w972) -> ("error out"=w974:errorcluster)  [unwired: 6 in, 1 out]
        n320 = call-poly "Enqueue Message.vi"("error in (no error)"=w974, "Message"="WaterFlowStartZeroLDO", "Message Queue"=w971) -> ("error out"=w975:errorcluster)  [unwired: 7 in, 1 out]
      }
      frame "WaterFlowPropOpenFVIR" {
        # "Start - Enable/Disable buttons appropriately for an acquisition that has started, and update status display."
        n321 = call-poly "Enqueue Message.vi"("error in (no error)"=w985, "Message Data"="Operator clicked on: Water Outlet Flow Proportional EPV-312B Open FVIR" ("Acquiring and Logging..."), "Message"="Update Status - FVIR", "Message Queue"=w984) -> ("error out"=w986:errorcluster)  [unwired: 6 in, 1 out]
        n322 = call-poly "Enqueue Message.vi"("error in (no error)"=w986, "Message"="WaterFlowPropOpenFVIR", "Message Queue"=w983) -> ("error out"=w987:errorcluster)  [unwired: 7 in, 1 out]
      }
      frame "WaterFlowPropOpenLDO" {
        # "Start - Enable/Disable buttons appropriately for an acquisition that has started, and update status display."
        n323 = call-poly "Enqueue Message.vi"("error in (no error)"=w997, "Message Data"="Operator clicked on: Water Outlet Flow Proportional EPV-312B Open LDO" ("Acquiring and Logging..."), "Message"="Update Status - LDO", "Message Queue"=w996) -> ("error out"=w998:errorcluster)  [unwired: 6 in, 1 out]
        n324 = call-poly "Enqueue Message.vi"("error in (no error)"=w998, "Message"="WaterFlowPropOpenLDO", "Message Queue"=w995) -> ("error out"=w999:errorcluster)  [unwired: 7 in, 1 out]
      }
      frame "WaterFlowPropCloseFVIR" {
        # "Start - Enable/Disable buttons appropriately for an acquisition that has started, and update status display."
        n325 = call-poly "Enqueue Message.vi"("error in (no error)"=w1009, "Message Data"="Operator clicked on: Water Outlet Flow Proportional EPV-312B Close FVIR" ("Acquiring and Logging..."), "Message"="Update Status - FVIR", "Message Queue"=w1008) -> ("error out"=w1010:errorcluster)  [unwired: 6 in, 1 out]
        n326 = call-poly "Enqueue Message.vi"("error in (no error)"=w1010, "Message"="WaterFlowPropCloseFVIR", "Message Queue"=w1007) -> ("error out"=w1011:errorcluster)  [unwired: 7 in, 1 out]
      }
      frame "WaterFlowPropCloseLDO" {
        # "Start - Enable/Disable buttons appropriately for an acquisition that has started, and update status display."
        n327 = call-poly "Enqueue Message.vi"("error in (no error)"=w1021, "Message Data"="Operator clicked on: Water Outlet Flow Proportional EPV-312B Close LDO" ("Acquiring and Logging..."), "Message"="Update Status - LDO", "Message Queue"=w1020) -> ("error out"=w1022:errorcluster)  [unwired: 6 in, 1 out]
        n328 = call-poly "Enqueue Message.vi"("error in (no error)"=w1022, "Message"="WaterFlowPropCloseLDO", "Message Queue"=w1019) -> ("error out"=w1023:errorcluster)  [unwired: 7 in, 1 out]
      }
      frame "WaterFlowStopLDO" {
        n329 = call-poly "Enqueue Message.vi"("error in (no error)"=w1030, "Message Data"="Operator clicked on: Water Flow Intellifaucet DRK375 Stop" ("Acquiring and Logging..."), "Message"="Update Status - LDO", "Message Queue"=w1027) -> ("error out"=w1034:errorcluster)  [unwired: 6 in, 1 out]
        n330 = call-poly "Enqueue Message.vi"("error in (no error)"=w1034, "Message"="WaterFlowStopLDO", "Message Queue"=w1028) -> ("error out"=w1029:errorcluster)  [unwired: 7 in, 1 out]
      }
      frame "WaterFlowStopZeroLDO" {
        n331 = call-poly "Enqueue Message.vi"("error in (no error)"=w1042, "Message Data"="Operator clicked on: Water Flow Intellifaucet DRK375 Stop" ("Acquiring and Logging..."), "Message"="Update Status - LDO", "Message Queue"=w1039) -> ("error out"=w1046:errorcluster)  [unwired: 6 in, 1 out]
        n332 = call-poly "Enqueue Message.vi"("error in (no error)"=w1046, "Message"="WaterFlowStopZeroLDO", "Message Queue"=w1040) -> ("error out"=w1041:errorcluster)  [unwired: 7 in, 1 out]
      }
      frame "OilSpray08Open" {
        # "Start - Enable/Disable buttons appropriately for an acquisition that has started, and update status display."
        n333 = call-poly "Enqueue Message.vi"("error in (no error)"=w1057, "Message Data"="Operator clicked on: Oil Spray 0.8 cc/min Open" ("Acquiring and Logging..."), "Message"="Update Status - LDO", "Message Queue"=w1056) -> ("error out"=w1058:errorcluster)  [unwired: 6 in, 1 out]
        n334 = call-poly "Enqueue Message.vi"("error in (no error)"=w1058, "Message"="OilSpray08Open", "Message Queue"=w1051) -> ("error out"=w1059:errorcluster)  [unwired: 7 in, 1 out]
      }
      frame "OilSpray08Close" {
        # "Start - Enable/Disable buttons appropriately for an acquisition that has started, and update status display."
        n335 = call-poly "Enqueue Message.vi"("error in (no error)"=w1069, "Message Data"="Operator clicked on: Oil Spray 0.8 cc/min Close" ("Acquiring and Logging..."), "Message"="Update Status - LDO", "Message Queue"=w1068) -> ("error out"=w1070:errorcluster)  [unwired: 6 in, 1 out]
        n336 = call-poly "Enqueue Message.vi"("error in (no error)"=w1070, "Message"="OilSpray08Close", "Message Queue"=w1063) -> ("error out"=w1071:errorcluster)  [unwired: 7 in, 1 out]
      }
      frame "OilSpray11Open" {
        # "Start - Enable/Disable buttons appropriately for an acquisition that has started, and update status display."
        n337 = call-poly "Enqueue Message.vi"("error in (no error)"=w1081, "Message Data"="Operator clicked on: Oil Spray 1.1 cc/min Open" ("Acquiring and Logging..."), "Message"="Update Status - LDO", "Message Queue"=w1080) -> ("error out"=w1082:errorcluster)  [unwired: 6 in, 1 out]
        n338 = call-poly "Enqueue Message.vi"("error in (no error)"=w1082, "Message"="OilSpray11Open", "Message Queue"=w1075) -> ("error out"=w1083:errorcluster)  [unwired: 7 in, 1 out]
      }
      frame "OilSpray11Close" {
        # "Start - Enable/Disable buttons appropriately for an acquisition that has started, and update status display."
        n339 = call-poly "Enqueue Message.vi"("error in (no error)"=w1093, "Message Data"="Operator clicked on: Oil Spray 1.1 cc/min Close" ("Acquiring and Logging..."), "Message"="Update Status - LDO", "Message Queue"=w1092) -> ("error out"=w1094:errorcluster)  [unwired: 6 in, 1 out]
        n340 = call-poly "Enqueue Message.vi"("error in (no error)"=w1094, "Message"="OilSpray11Close", "Message Queue"=w1087) -> ("error out"=w1095:errorcluster)  [unwired: 7 in, 1 out]
      }
      frame "OilSpray133Open" {
        # "Not used right now."
        # "Start - Enable/Disable buttons appropriately for an acquisition that has started, and update status display."
        n341 = call-poly "Enqueue Message.vi"("error in (no error)"=w1105, "Message Data"="Operator clicked on: Oil Spray 1.33 cc/min Open" ("Acquiring and Logging..."), "Message"="Update Status - LDO", "Message Queue"=w1104) -> ("error out"=w1106:errorcluster)  [unwired: 6 in, 1 out]
        n342 = call-poly "Enqueue Message.vi"("error in (no error)"=w1106, "Message"="OilSpray133Open", "Message Queue"=w1099) -> ("error out"=w1107:errorcluster)  [unwired: 7 in, 1 out]
      }
      frame "OilSpray133Close" {
        # "Start - Enable/Disable buttons appropriately for an acquisition that has started, and update status display."
        n343 = call-poly "Enqueue Message.vi"("error in (no error)"=w1117, "Message Data"="Operator clicked on: Oil Spray 1.33 cc/min Close" ("Acquiring and Logging..."), "Message"="Update Status - LDO", "Message Queue"=w1116) -> ("error out"=w1118:errorcluster)  [unwired: 6 in, 1 out]
        n344 = call-poly "Enqueue Message.vi"("error in (no error)"=w1118, "Message"="OilSpray133Close", "Message Queue"=w1111) -> ("error out"=w1119:errorcluster)  [unwired: 7 in, 1 out]
      }
      frame "HeaterON" {
        # "Start - Enable/Disable buttons appropriately for an acquisition that has started, and update status display."
        n345 = call-poly "Enqueue Message.vi"("error in (no error)"=w1129, "Message Data"="Operator clicked on: Heater ON..." ("Acquiring and Logging..."), "Message"="Update Status - LDO", "Message Queue"=w1128) -> ("error out"=w1130:errorcluster)  [unwired: 6 in, 1 out]
        n346 = call-poly "Enqueue Message.vi"("error in (no error)"=w1130, "Message"="HeaterON", "Message Queue"=w1127) -> ("error out"=w1131:errorcluster)  [unwired: 7 in, 1 out]
      }
      frame "HeaterOFF" {
        # "Start - Enable/Disable buttons appropriately for an acquisition that has started, and update status display."
        n347 = call-poly "Enqueue Message.vi"("error in (no error)"=w1141, "Message Data"="Operator clicked on: Heater OFF..." ("Acquiring and Logging..."), "Message"="Update Status - LDO", "Message Queue"=w1140) -> ("error out"=w1142:errorcluster)  [unwired: 6 in, 1 out]
        n348 = call-poly "Enqueue Message.vi"("error in (no error)"=w1142, "Message"="HeaterOFF", "Message Queue"=w1139) -> ("error out"=w1143:errorcluster)  [unwired: 7 in, 1 out]
      }
      frame "SendParamToPLCFVIR" {
        # "Start - Enable/Disable buttons appropriately for an acquisition that has started, and update status display."
        n349 = call-poly "Enqueue Message.vi"("error in (no error)"=w1159, "Message Data"="Operator clicked on: Send parameters to PLC FVIR ..." ("Acquiring and Logging..."), "Message"="Update Status - FVIR", "Message Queue"=w1158) -> ("error out"=w1160:errorcluster)  [unwired: 6 in, 1 out]
        n350 = Build Array("Time Delay of Change direction of Mannequin Actuators", "Number of Mannequin Movement", "Water Outlet Proportional Valve EPV-312B", "Water Temperature Intellifaucet DRK375", "Water Flow Intellifaucet DRK375", "Time Pause Between Next Mannequin Sequence") -> (w1149:u16[])
        n351 = call-poly "Enqueue Message.vi"("error in (no error)"=w1160, "Message Data"=w1149, "Message"="SendParamToPLCFVIR", "Message Queue"=w1157) -> ("error out"=w1161:errorcluster)  [unwired: 6 in, 1 out]
      }
      frame "SendParamToPLCLDO" {
        # "Start - Enable/Disable buttons appropriately for an acquisition that has started, and update status display."
        n352 = call-poly "Enqueue Message.vi"("error in (no error)"=w1198, "Message Data"="Operator clicked on: Send parameters to PLC LDO ..." ("Acquiring and Logging..."), "Message"="Update Status - LDO", "Message Queue"=w1197) -> ("error out"=w1199:errorcluster)  [unwired: 6 in, 1 out]
        n353 = Build Array("Burner cycle 1 to 10 - Duty cycle ON (default 55 min.)", "Burner cycle 1 to 10 - Duty cycle OFF (default 5 min.)", "Burner cycle 11 to 12 - Duty cycle ON (default 235 min.)", "Burner cycle 11 to 12 - Duty cycle OFF (default 5 min.)", "Burner cycle 13 to end - Duty cycle ON (default 55 min.)", "Burner cycle 13 to end - Duty cycle OFF (default 5 min.)", "Oil 1st sequence ON (default 5 min.)", "Oil 1st sequence OFF (default 5 min.)", "All subsequent sequence ON (default 3 min.)", "All subsequent sequence OFF (default 27 min.)", "Oil spray preconditioning period ON (default 10 min.)", "Oil spray preconditioning period OFF  (default 20 min.)", "Precondition Purge Gallons") -> (w1194:u16[])
        n354 = call-poly "Enqueue Message.vi"("error in (no error)"=w1199, "Message Data"=w1194, "Message"="SendParamToPLCLDO", "Message Queue"=w1196) -> ("error out"=w1178:errorcluster, "dup Message Queue"=w1179:refnum<queue>)  [unwired: 6 in]
        n355 = case shown="False" "Temp/Flow PID Selector" {
          tunnel: ["PID_Selector_OFF" "PID_Selector_ON"] -> w1164
          frame False {
          }
          frame True {
          }
        }
        n356 = call-poly "Enqueue Message.vi"("error in (no error)"=w1178, "Message Data"="Output Temperature Target (Automated Test)", "Message"="Output_Temperature_Target", "Message Queue"=w1179) -> ("error out"=w1172:errorcluster, "dup Message Queue"=w1171:refnum<queue>)  [unwired: 6 in]
        n357 = call-poly "Enqueue Message.vi"("error in (no error)"=w1172, "Message Data"="Output Flow Rate Target (Automated Test)", "Message"="Output_Flow_Target", "Message Queue"=w1171) -> ("error out"=w1168:errorcluster, "dup Message Queue"=w1166:refnum<queue>)  [unwired: 6 in]
        n358 = call-poly "Enqueue Message.vi"("error in (no error)"=w1168, "Message"=w1164, "Message Queue"=w1166) -> ("error out"=w1167:errorcluster)  [unwired: 7 in, 1 out]
      }
      frame "DataToShow" {
        # "FVIR block sends out boolean if one of the 4 tubes are >= 1.8"
        # "If one of the 4 tubes for % Butane are >= 1.8, the test will stop"
        # "Update Status - Convert the message data to a string to display in the Status indicator."
        n359 = Variant To Data(error in=w1217, type=string[] [], Variant=w1216) -> (data=w1212:string[], error out=w1211:errorcluster)
        n360 = call "DisplayTemperaturesFVIR.vi"("Array"=w1212) -> ("FVIR array 2"=→"Temperatures - FVIR":string[][], "Logical OR array"=w1207:bool)  [unwired: 8 in]
        n361 = case shown="True" w1207 {
          tunnel: w1211 -> [w1220 w1225]
          tunnel: [w1220 w1224] -> w1210
          tunnel: w1209 -> [_ w1223]
          tunnel: w1208 -> [w1219 w1222]
          tunnel: [w1219 w1221] -> w1206
          frame False {
          }
          frame True {
            n362 = case shown="False" w1222 {
              tunnel: w1225 -> [w1227 w1232]
              tunnel: [w1227 w1231] -> w1224
              tunnel: w1223 -> [_ w1230]
              tunnel: [TRUE ("new element/subarray") TRUE ("new element/subarray")] -> w1221
              frame True {
              }
              frame False {
                n363 = call-poly "Enqueue Message.vi"("error in (no error)"=w1232, "Message"="StopTestCaseFVIR", "Message Queue"=w1230) -> ("error out"=w1231:errorcluster)  [unwired: 7 in, 1 out]
              }
            }
          }
        }
        "Higher than 1.8% butane" <- w1206
        n364 = Merge Errors(w1210) -> (w1218:errorcluster)
      }
      frame "DisplayAllData" {
        w1259 = 0.0 ("HHV_1")
        # "Only for LDO...need to add FVIR"
        # "Write the string"
        n365 = Unbundle By Name(w1238) -> ("PLC Data Out"=w1260:T3)
        n366 = Unbundle By Name(w1238) -> ("PLC Data Out.LDO Control Input.Sensor Data"=w1256:string[][], "Gas Data.Data Cluster"=w1258:T8, "Gas Data.Header Array"=w1257:string[], "Inficon Data Input.Gross Heating Value, Vol (Real, Dry)"=w1254:dbl, "Ultramat 23"=w1234:string[][], "PLC Data Out.LDO Control Input"=w1235:T5)
        n367 = Unbundle By Name(w1260) -> ("FVIR Data Input.FVIR PLC lifebit"=→"FVIR PLC lifebit":bool, "FVIR Data Input.Mannequin is moving - FVIR"=→"Mannequin is moving - FVIR":bool, "FVIR Data Input.Can is spilling - FVIR"=→"Can is spilling - FVIR":bool, "FVIR Data Input.Water Outlet Valve - FVIR"=→"Water Outlet Valve - FVIR":bool, "FVIR Data Input.Water Inlet Valve - FVIR"=→"Water Inlet Valve - FVIR":bool, "FVIR Data Input.Gas Solenoid Valve - FVIR"=→"Gas Solenoid Valuce - FVIR":bool, "FVIR Data Input.Water flow DRK375 is open - FVIR"=→"Water flow DRK375 is open - FVIR":bool, "FVIR Data Input.Actuator mannequin is going to Home Pos - FVIR"=→"Actuator mannequin is going to Home Pos - FVIR":bool, "FVIR Data Input.Actuator mannequin is going to Work Pos - FVIR"=→"Actuator mannequin is going to Work Pos - FVIR":bool, "FVIR Data Input.Actuator spill can is going to Home Pos - FVIR"=→"Actuator spill can is going to Home Pos - FVIR":bool, "FVIR Data Input.Actuator spill can is going to Work Pos - FVIR"=→"Actuator spill can is going to Work Pos - FVIR":bool, "FVIR Data Input.Start recording data - FVIR"=→"Start recording data - FVIR":bool, "FVIR Data Input.Status for Error - FVIR"=→"Status for error - FVIR":string, "FVIR Data Input.Error-FVIR"=→"Error - FVIR":bool, "FVIR Data Input.Sensors -FVIR"=→"Sensors - FVIR":string[][], "FVIR Data Input.Water Outlet Flow Proportional - FVIR"=→"Water Outlet Flow Proportional - FVIR":bool, "FVIR Data Input.Test chamber is in sequence - FVIR"=→"Test chamber is in sequence - FVIR":bool)
        n368 = Unbundle By Name(w1260) -> ("LDO Control Input.Start recording data - LDO"=→"Start recording data - LDO":bool, "LDO Control Input.Water Outlet Valve - LDO"=→"Water Outlet Valve - LDO":bool, "LDO Control Input.Water Inlet Valve - LDO"=→"Water Inlet Valve - LDO":bool, "LDO Control Input.Gas Solenoid Valve - LDO"=→"Gas Solenoid Valuce - LDO":bool, "LDO Control Input.Water flow DRK375 is open - LDO"=→"Water flow DRK375 is open - LDO":bool, "LDO Control Input.Oil spray 0.8cc/min - LDO"=w1244:bool, "LDO Control Input.Oil spray 1.1cc/min - LDO"=w1243:bool, "LDO Control Input.Oil spray 1.33cc/min - LDO"=w1242:bool, "LDO Control Input.Heater ON/OFF - LDO"=→"Heater ON/OFF - LDO":bool, "LDO Control Input.Water Outlet Flow Proportional - LDO"=→"Water Outlet Flow Proportional - LDO":bool, "LDO Control Input.Status for error - LDO"=→"Status for error - LDO":string, "LDO Control Input.Error - LDO"=→"Error - LDO":bool, "LDO Control Input.Test chamber is in sequence - LDO"=→"Test chamber is in sequence - LDO":bool)
        "Oil spray 1.33cc/min - LDO" <- w1242
        "Oil spray 1.1cc/min - LDO" <- w1243
        "Oil spray 0.8cc/min - LDO" <- w1244
        n369 = call "LDO Bit Status Write.vi"("LDO Control Input"=w1235) -> ("Bit Status"=w1233:string[][])  [unwired: 9 in, 1 out]
        n370 = call "Write String Array Units.vi"("Total_1"=w1259, "HHV_1"=w1259, "Error In"=w1253, "Gross Heating Value, Vol (Real, Dry)"=w1254, "Header Array"=w1257, "Data Cluster"=w1258) -> ("Error Out"=w1250:errorcluster, "Gas Rate (BTU/hr)"=w1252:dbl, "String Data"=w1255:string[][])  [unwired: 3 in]
        n371 = Build Array (concatenate)(w1256, w1255, w1234, w1233) -> (w1236:string[][])
        "Data" <- w1236
        n372 = Bundle By Name(cluster=w1238, "PLC Data Out.Data to Save.LDO Full Data"=w1236) -> (w1237:T2)
        n373 = control-ref of="Burner ON"() -> (w1249:refnum<vi>)
        n374 = control-ref of="Oil spray 0.8cc/min - LDO"() -> (w1248:refnum<vi>)
        n375 = control-ref of="Oil spray 1.1cc/min - LDO"() -> (w1247:refnum<vi>)
        n376 = control-ref of="Oil spray 1.33cc/min - LDO"() -> (w1246:refnum<vi>)
        n377 = Greater?(x=w1252, y="Pilot Rate (BTU/hr)") -> (0:w1241:bool)
        n378 = call "LDO Trigger Events.vi"("Event Booleans in"=w1245, "Burner ON Ref"=w1249, "0.8 ML Ref"=w1248, "1.1 ML Ref"=w1247, "1.33 ML Ref"=w1246, "Oil spray 0.8cc/min - LDO"=w1244, "Burner ON"=w1241, "Oil spray 1.1cc/min - LDO"=w1243, "Oil spray 1.33cc/min - LDO"=w1242) -> ("Event Booleans out"=w1240:T1)  [unwired: 10 in]
        n379 = Unbundle By Name(w1240) -> ("Burner ON"=→"Burner ON":bool)
      }
      frame "DisplayValuesFromPLC" {
        # "Update Status - Convert the message data to a string to display in the Status indicator."
        n380 = Unbundle By Name(w1293) -> ("PLC Data Out"=w1294:T3)
        n381 = Variant To Data(error in=w1313, type=u16[] [1, 0, 0, 0, 0, 0, 0, 0] ("Input Registers"), Variant=w1312) -> (data=w1307:u16[], error out=w1306:errorcluster)
        n382 = call "DisplayValuesFromPLC.vi"("PLC Data"=w1294, "error in"=w1306, "Input Registers"=w1307) -> ("error out"=w1305:errorcluster, "PLC Data Out"=w1304:T3)  [unwired: 7 in]
        n383 = call "DisplayValuesFromPLC_LDO.vi"("error in"=w1305, "PLC Data"=w1304) -> ("error out"=w1300:errorcluster, "PLC Data Out"=w1302:T3)  [unwired: 8 in]
        n384 = call "FVIR Button Disable.vi"("UI Refs"=w1303, "error in (no error)"=w1300, "PLC Data In"=w1302, "Queue in"=w1310) -> ("error out"=w1299:errorcluster, "PLC Data Out"=w1301:T3, "Queue out"=w1309:refnum<queue>)  [unwired: 5 in]
        n385 = call "LDO Button Disable.vi"("UI Refs"=w1303, "error in (no error)"=w1299, "PLC Data In"=w1301, "Queue in"=w1309) -> ("error out"=w1296:errorcluster, "PLC Data Out"=w1292:T3, "dup Message Queue"=w1297:refnum<queue>)  [unwired: 5 in]
        n386 = call-poly "Enqueue Message.vi"("error in (no error)"=w1296, "Message"="DisplayAllData", "Message Queue"=w1297) -> ("error out"=w1295:errorcluster)  [unwired: 7 in, 1 out]
        n387 = Bundle By Name(cluster=w1293, "PLC Data Out"=w1292) -> (w1291:T2)
      }
      frame "DisplayValuesFromAlicat_LDO" {
        n388 = Variant To Data(error in=w1324, type=T7 {"Data Cluster"={"Absolute Pressure"=0.0, "Gauge/Diff. Pressure"=0.0, "Barometric Pressure"=0.0, "Temperature"=0.0, "Volumetric Flow"=0.0, "Mass Flow"=0.0, "Setpoint"=0.0, "Valve Drive"=0.0, "Totalizer"=0.0, "[hr]"=0.0, "[min]"=0.0, "[sec]"=0.0, "Totalizer Average Flow"=0.0, "Totalizer Peak Flow"=0.0, "Gas selected"=""}, "Units of Measure Input"={"Abs. Pressure"="", "Gauge/Diff. Press."="", "Barometric Press."="", "Temperature"="", "Volume"="", "Mass"="", "Setpoint"="", "Valve Drive"="", "Totalizer"="", "Tot. Timer"="", "Tot. Avg. Flow"="", "Tot. Peak Flow"=""}, "Header Array"=[]} ("Gas Data"), Variant=w1323) -> (data=w1315:T7, error out=w1320:errorcluster)
        n389 = Bundle By Name(cluster=w1317, "Gas Data"=w1315) -> (w1316:T2)
        n390 = call-poly "Enqueue Message.vi"("error in (no error)"=w1320, "Message"="DisplayAllData", "Message Queue"=w1321) -> ("error out"=w1319:errorcluster)  [unwired: 7 in, 1 out]
      }
      frame "DisplayValuesFromInficon" {
        w1336 = T10 {"Gross Heating Value, Vol (Real, Dry)"=0.0, "Nitrogen Component Normalized Mole % (Dry)"=0.0, "Methane Component Normalized Mole % (Dry)"=0.0, "Carbon Dioxide Component Normalized Mole % (Dry)"=0.0, "Ethane Component Normalized Mole % (Dry)"=0.0, "Propane Component Normalized Mole % (Dry)"=0.0, "i-Pentane Component Normalized Mole % (Dry)"=0.0, "i-Butane Component Normalized Mole % (Dry)"=0.0, "n-Butane Component Normalized Mole % (Dry)"=0.0, "n-Pentane Component Normalized Mole % (Dry)"=0.0, "Hexane Component Normalized Mole % (Dry)"=0.0, "Heptane Component Normalized Mole % (Dry)"=0.0, "Gross Wobbe Index, Real(Dry)"=0.0, "Relative Density, Real(Dry)"=0.0, "Propylene Component Normalized Mole % (Dry)"=0.0, "C4 Olefins Component Normalized Mole % (Dry)"=0.0, "Water Component Normalized Mole % (Dry)"=0.0}  # Inficon Data Input
        n391 = Variant To Data(error in=w1337, type=w1336, Variant=w1335) -> (data=w1328:T10, error out=w1333:errorcluster)
        n392 = Bundle By Name(cluster=w1330, "Inficon Data Input"=w1328) -> (w1329:T2)
        n393 = call-poly "Enqueue Message.vi"("error in (no error)"=w1333, "Message"="DisplayAllData", "Message Queue"=w1331) -> ("error out"=w1332:errorcluster)  [unwired: 7 in, 1 out]
      }
      frame "DisplayValuesFromUltramat" {
        n394 = Variant To Data(error in=w1350, type=string[][] [], Variant=w1349) -> (data=w1341:string[][], error out=w1347:errorcluster)
        n395 = Bundle By Name(cluster=w1344, "Ultramat 23"=w1341) -> (w1343:T2)
        n396 = call-poly "Enqueue Message.vi"("error in (no error)"=w1347, "Message"="DisplayAllData", "Message Queue"=w1345) -> ("error out"=w1346:errorcluster)  [unwired: 7 in, 1 out]
      }
      frame "CheckBeforeWriteDataLDO" {
        n397 = Unbundle By Name(w1354) -> ("PLC Data Out"=w1353:T3)
        n398 = call-poly "Enqueue Message.vi"("error in (no error)"=w1358, "Message Data"=w1353, "Message"="CheckBeforeWriteDataLDO", "Message Queue"=w1356) -> ("error out"=w1357:errorcluster)  [unwired: 6 in, 1 out]
      }
      frame "CheckBeforeWriteDataFVIR" {
        n399 = Unbundle By Name(w1363) -> ("PLC Data Out"=w1362:T3)
        n400 = call-poly "Enqueue Message.vi"("error in (no error)"=w1367, "Message Data"=w1362, "Message"="CheckBeforeWriteDataFVIR", "Message Queue"=w1365) -> ("error out"=w1366:errorcluster)  [unwired: 6 in, 1 out]
      }
      frame "Error" {
        # "Error - Display an error dialog. This message is sent by the \"Error Handler\" VIs at the end of other loops in this application."
        n401 = Variant To Data(error in=w1374, type=errorcluster {"status"=FALSE, "code"=0, "source"=""} ("error constant"), Variant=w1377) -> (data=w1375:errorcluster, error out=w1378:errorcluster)
        n402 = call <vilib>:"Simple Error Handler.vi"("error in (no error)"=w1375) -> ()  [unwired: 4 in, 5 out]
        n403 = Merge Errors(w1378) -> (w1376:errorcluster)
      }
      frame "Exit" {
        w1384 = TRUE ("Priority Message? (F)")
        w1382 = "Exit" ("Message")
        # "Popup an error dialog if 'Exit' was called as a result of an error."
        # "Stop the VI"
        # "Exit - Send Exit messages to the Acquisition and Logging loops, and fire the user event to stop the Event Handling Loop."
        n404 = Variant To Data(type=errorcluster {"status"=FALSE, "code"=0, "source"=""} ("error constant"), Variant=w1402) -> (data=w1401:errorcluster)  [unwired: 1 in, 1 out]
        n405 = call <vilib>:"Simple Error Handler.vi"("error in (no error)"=w1401) -> ()  [unwired: 4 in, 5 out]
        n406 = call-poly "Enqueue Message.vi"("Priority Message? (F)"=w1384, "error in (no error)"=w1394, "Message"=w1382, "Message Queue"=w1400) -> ("error out"=w1399:errorcluster)  [unwired: 6 in, 1 out]
        n407 = call-poly "Enqueue Message.vi"("Priority Message? (F)"=w1384, "error in (no error)"=w1399, "Message"=w1382, "Message Queue"=w1398) -> ("error out"=w1397:errorcluster)  [unwired: 6 in, 1 out]
        n408 = call-poly "Enqueue Message.vi"("Priority Message? (F)"=w1384, "error in (no error)"=w1397, "Message"=w1382, "Message Queue"=w1396) -> ("error out"=w1393:errorcluster)  [unwired: 6 in, 1 out]
        n409 = call-poly "Enqueue Message.vi"("Priority Message? (F)"=w1384, "error in (no error)"=w1393, "Message"=w1382, "Message Queue"=w1392) -> ("error out"=w1391:errorcluster)  [unwired: 6 in, 1 out]
        n410 = call-poly "Enqueue Message.vi"("Priority Message? (F)"=w1384, "error in (no error)"=w1391, "Message"=w1382, "Message Queue"=w1390) -> ("error out"=w1388:errorcluster)  [unwired: 6 in, 1 out]
        n411 = call-poly "Enqueue Message.vi"("Priority Message? (F)"=w1384, "error in (no error)"=w1388, "Message"=w1382, "Message Queue"=w1387) -> ("error out"=w1386:errorcluster)  [unwired: 6 in, 1 out]
        n412 = call-poly "Enqueue Message.vi"("Priority Message? (F)"=w1384, "error in (no error)"=w1386, "Message"=w1382, "Message Queue"=w1383) -> ("error out"=w1385:errorcluster)  [unwired: 6 in, 1 out]
        n413 = call "Fire User Event - Stop.vi"("error in (no error)"=w1385, "User Event - Stop"=w1406) -> ("error out"=w1405:errorcluster)  [unwired: 9 in]
      }
      frame "---Copy This Frame---" {
        # "Duplicate this frame when creating new messages.  Change this comment in the duplicated frame to describe this message."
        n414 = Merge Errors(w1413) -> (w1412:errorcluster)
      }
      frame Default {
        # "'Default' case only runs if there is a message that isn't defined in any of the other cases.  Output a programming error."
        n415 = xnode "Error Ring"("parameter 0"=w1418) -> ("error out"=w1417:errorcluster)
      }
    }
    n416 = disable-structure shown="Disabled" {
      disable-tunnel: w347 -> [w375 w376]
      disable-tunnel: w346 -> [w374 _]
      disable-tunnel: [w373 w376] -> w345
      frame Disabled {
        n417 = Build Array (concatenate)(w375, w374) -> (w373:string[])
        "Message Loop" <- w373
      }
      frame Enabled {
      }
    }
    n418 = call "Error Handler - Message Handling Loop.vi"("error in (no error)"=w363, "Message Queue"=w362) -> ("dup error in"=w364:errorcluster)  [unwired: 8 in, 1 out]
    "Numeric" <- w350
  }
  n419 = Unregister For Events(event registration refnum=w32, error in=w35) -> (error out=w33:errorcluster)
  n420 = Release Queue(queue=w19, error in (no error)=w36) -> (error out=w20:errorcluster)  [unwired: 1 in, 2 out]
  n421 = Merge Errors(w33, w20, w23, w22, w21, w18, w9, w8, w7) -> (w30:errorcluster)
  n422 = call "Destroy User Event - Stop.vi"("error in (no error)"=w30, "User Event - Stop"=w26) -> ("error out"=w29:errorcluster)  [unwired: 9 in]
  n423 = disable-structure shown="Default" {
    disable-tunnel: w29 -> [_ _]
    frame condition #0 (active) {
    }
    frame condition #1 {
      # "Call Quit LabVIEW if running as a built application."
      n424 = Quit LabVIEW() -> ()  [unwired: 1 in]
    }
  }
